vi "Dashboard Main.vi"() -> ()   [LabVIEW 2015]
uses:
  Camera Types.ctl
  <vilib>/Utility/miscctls.llb/LVRowAndColumnTypeDef.ctl
  <vilib>/event_ctls.llb/eventvkey.ctl
  <vilib>/Rock Robotics/WPI/Dashboard/WPI_DashboardLogging Global.vi
  <vilib>/Rock Robotics/Network Tables/NT Read Boolean.vi
  <vilib>/Utility/config.llb/Write Key (String).vi
  <vilib>/Utility/config.llb/Write Key (I32).vi
  <vilib>/Utility/config.llb/NI_LVConfig.lvlib
panel:
  in  "Input 2":u32
  in  "Input 1":u32
  out "Shooter Position":dbl
  out "Stowed Indicator":bool=TRUE
  out "Barf Shot Indicator":bool
  out "Far Shot Indicator":bool
  out "Close Shot Indicator":bool caption="Shooter Position"
  out "Yaw Indicator":bool
  out "Target Indicator":bool=TRUE
  out "Distance Indicator":bool=TRUE
  out "Angle Indicator":bool
  out "Ball Present Indicator":bool
  in  "TCP":refnum<k5>
  out "Camera IP":string="169.254.26.48"
  out "Image Message":string="Timeout in Camera Communications"
  in  "Dashboard Tab":T1(tab)=enum."Configuration"
  in  "Test Slider":dbl(slide) scale=0.0..100.0 scale format="%#_3g"
  in  "On/Off":bool caption="Solenoid"
  in  "Test Name":u16(ring) items=["Select the test to run..."]
  in  "Test Tree":string(tree)
  in  "Motor":cluster{"Value":dbl, "Enable":bool} {"Value" scale=-1.0..1.0 scale format="%#_3g"}
  out "Progress":T2 {"Test Progress" scale=0.0..100.0}
  in  "Rev/Fwd":cluster{"Forward":bool, "Reverse":bool}
  in  "Test Ring":u16(ring) items=["Monochrome", "Color"]
  out "Cmd Status":string
  in  "Execute Command":bool
  in  "Command Params":string[][](table)=[["No Input Parameters", "", ""]]
  in  "Command Selection":i32(listbox)
  in  "CheckList":i32(listbox)
  out "Tree":string(tree)
  in  "Tab Control":T3(tab)=enum."Load / Save"
  in  "Autonomous Mode":enum32{"0", "1", "2", "3"}(ring)
  in  "Position":i32(slide)=1 min=1 max=5 step=1 scale=1.0..5.0
  in  "Calibrate":bool
  out "Highest Score":dbl
  out "Distance (ft)":dbl
  in  "Reflective Tape Color":T4={"Hue"={112.792542, 147.565674}, "Sat"={128.447754, 128.447754}, "Val"={63.844784, 227.916416}} caption="Color Components" {"Val" scale=0.0..255.0; "Sat" scale=0.0..255.0; "Hue" scale=0.0..255.0 scale format="%#_3g"}
  in  "Test Mode":bool
  in  "Image":dbl=2.0 min=1.0 max=12.0 step=1.0
  in  "Min Score":dbl(slide) min=0.0 max=100.0 step=1.0 scale=0.0..100.0 scale format="%d%%"
  in  "Camera":T5=enum."MS HD3000 square"
  out "Targets":i32
  out "Vision Target Center":dbl=160.0 caption="Center (px)"
  in  "Y 2":dbl=60.0
  in  "X 2":dbl=100.0
  in  "Thickness 2":dbl=2.0
  in  "Y 1":dbl(slide)=126.0 scale=0.0..250.0
  in  "X 1":dbl(slide)=169.290323 scale=0.0..320.0
  in  "Show Center Line":bool
  in  "Close Shot Distance (ft)":dbl(slide)=9.0 min=0.0 max=10.0 scale=0.0..10.0
  in  "Far Shot Distance (ft)":dbl(slide)=10.5 min=0.0 max=10.0 scale=0.0..10.0
  in  "Close Shot":u32(colorbox)=16769066
  in  "Far Shot":u32(colorbox)=3538688
  in  "Show Target Box":bool=TRUE
  in  "Text Size":dbl
  in  "Too Far":u32(colorbox)=15663156
  in  "Show Crosshairs":bool=TRUE
  in  "Thickness 1":dbl=2.0
  out "Drivetrain Test Enabled":bool
  in  "D":dbl
  in  "I":dbl
  in  "P":dbl
  in  "Apply Test PID Values":bool
  in  "Px/Deg Conversion":dbl=0.1825 caption="1 px =                  degrees" min=0.0
  out "Difference (px)":dbl=-157.5
  out "Robot Center":dbl=317.5
  out "Target Align Center":dbl=160.0 caption="Target Center"
  out "Target Align Yaw Indicator":cluster{dbl, dbl}(knob) scale=-180.0..180.0
  out "Status":string
  out "INI File Path":path=path "Documents/FRC/DashboardSettings.ini"
  in  "Save Settings":bool
  out "File Created":bool
  out "Difference":dbl
  out "Starting Position":i32
  out "Autonomous Mode":enum32{"0", "1", "2", "3"}(ring)
  out "Intake":cluster{dbl, dbl}(knob) scale=0.0..5.0
  out "Time Remaining":dbl(slide)=-1.0 scale=-1.0..135.0 scale format="%#_6f"
  out "Battery Voltage":dbl(slide)=12.73828125 scale=0.012..12.0 scale format="%#_6f"
  out "Shooter":cluster{dbl, dbl}(knob) scale=0.0..5.0
  out "Yaw":cluster{dbl, dbl}(knob) scale=-180.0..180.0
  out "NT Connection":bool=TRUE
  in  "Camera Settings":T6={"Frame Rate"=30, "Compression"=30, "Size"=1} {"Frame Rate" scale=1.0..30.0; "Size" items=["640x480", "320x240", "160x120"]}
  out "Mode":T7(ring)
  in  "DB Camera Config":bool
  out "fps":dbl=30.150753768844222 format="%#.1g"
  out "Mbps":dbl=4.785927884198665 format="%#.1g"
  out "Mbps LED":bool=TRUE
  in  "Vision":u16(ring)=2 items=["Camera Off", "USB Camera SW", "USB Camera HW", "IP Camera", "Local"]
  in  "Rec Mode":enum32{"Stop", "Record", "Playback"}(radio)
  out "Background":bool=TRUE
  out "Distance":dbl
  out "Camera Image":T8(plugin-control)
  # "Close Shot"
  # "Far Shot"
  # "Target Box"
  # "Drivetrain Test PID Values"
  # "deg/px"
  # "Current Yaw"
  # "Target Yaw"
  # "* deg/px doesn't get saved, just initialized as default value"
  # "Setpoint"
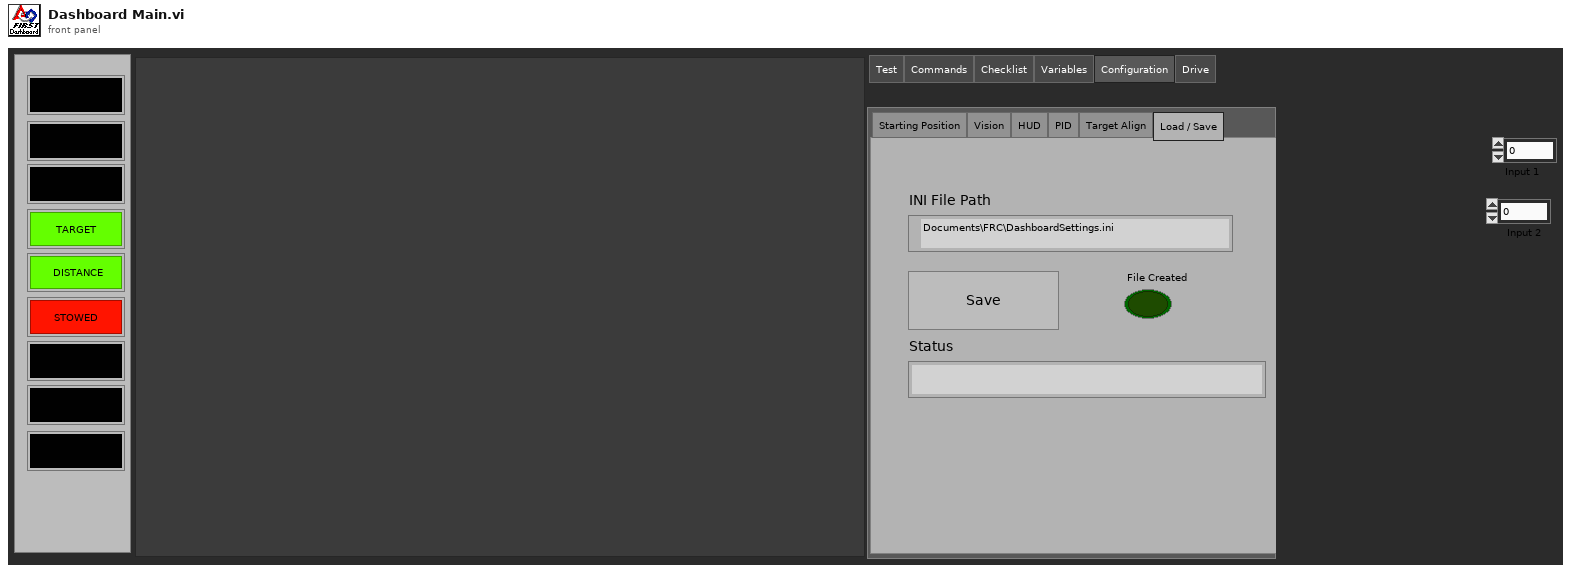
[diagram p1: front panel]
types:
  T1 = enum32{"Test", "Commands", "Checklist", "Variables", "Configuration", "Drive"}
  T2 = cluster{"Test Progress":u8, "Test Progress Text":string}
  T3 = enum32{"Starting Position", "Vision", "HUD", "PID", "Target Align", "Load / Save"}
  T4 = cluster{"Hue":cluster{dbl, dbl}, "Sat":cluster{dbl, dbl}, "Val":cluster{dbl, dbl}}
  T5 = typedef "Camera Types.ctl" = enum16{"206", "1011", "1013", "MS HD3000 square", "MS HD3000 640x480"}
  T6 = cluster{"Frame Rate":i32, "Compression":i32, "Size":u16}
  T7 = enum8{"Tele-Op Disabled", "Tele-Op Enabled", "Auto Disabled", "Auto Enabled", "Test Disabled", "Test Enabled", "Disconnected", "No Code", "E-Stop"}
  T8 = typedef "IMAQ Image.ctl" = refnum<image>
  T9 = typedef "Image Type" = u32
  T10 = cluster{"IDs":cluster{"RPC field ID":u16, "Unique ID":u16}, "String":string}
  T11 = cluster{"Camera Image":refnum<vi>, "Dashboard Tab":refnum<vi>, "Background":refnum<vi>, "Vision":refnum<vi>, "Rec Mode":refnum<vi>, "Test Slider":refnum<vi>, "On/Off ":refnum<vi>, "Test Ring":refnum<vi>, "Rev/Fwd":refnum<vi>, "Test Name":refnum<vi>, "Motor":refnum<vi>, "Progress":refnum<vi>, "CheckList":refnum<vi>, "Tree":refnum<vi>, "Test Tree":refnum<vi>, "Command Params":refnum<vi>, "Command Selection":refnum<vi>, "Execute Command":refnum<vi>, "Cmd Status":refnum<vi>}
  T12 = typedef "NI_LVConfig.lvlib/Config Data RefNum.ctl" = refnum<k1>
  T13 = cluster{"Error Strings":string, "Disable Counts":cluster{u16, u16}, "Rail Faults":cluster{u16, u16, u16}, "Robot IP":string, "DB Mode":u8, "Event Info":cluster{"Name":string, "Type":u8, "Number":u16, "Replay":u8}, "Camera Addr":string}
  T14 = cluster{"Storage":cluster{"Disk Free":u64, "RAM Block":u32, "RAM free":u32}, "CPU Utilization":cluster{"CPU % ISR":sgl, "CPU % Time Crit":sgl, "CPU % Timed Str":sgl, "CPU % High":sgl, "CPU % Above":sgl, "CPU % Normal":sgl, "CPU % Low":sgl}, "CAN":cluster{"% Bus Utilization":sgl, "Bus Off Cnt":u32, "TX_FIFO Full Cnt":u32, "Receive Error Cnt":u8, "Transmit Error Cnt":u8}, "HID":cluster{"HID Outputs":u32, "Rumble Low":u16, "Rumble High":u16}[]}
  T15 = cluster{"Status bits":cluster{"Test Mode":bool, "Autonomous":bool, "Enabled":bool, "Code Start":bool, "Brownout":bool, "Reserved 2":bool, "Reserved 3":bool, "E-Stop":bool}, "Code Trace":cluster{"Disabled":bool, "TeleOp":bool, "Auto":bool, "Test":bool}, "Controller Type":enum16{"unknown", "cRIO", "roboRio"}, "Code?":enum16{"unknown", "noCode", "code"}, "Battery V":dbl}
  T16 = cluster{"Control Bits":cluster{"TestMode":bool, "Autonomous":bool, "Enabled":bool, "FMS Present":bool, bool, bool, bool, "E-Stop":bool}, "Team Station ":u8, "Countdown":sgl, "Joystick Values":cluster{"Axes":dbl[], "Buttons":bool[], "POVs":i16[]}[]}
  T17 = cluster{"Operation":enum16{"Update", "Clear"}, "Color Box":u32}[]
  T18 = typedef "eventvkey.ctl" = enum16{"ASCII", "Enter", "Return", "Shift", "Ctrl", "Alt", "Cmd", "Opt", "Caps", "NumLock", "Clear", "Break", "Up", "Down", "Left", "Right", "Insert", "Delete", "Home", "End", "PageUp", "PageDown", "Escape", "Help", "Pause", "ScrollLock", "F1", "F2", "F3", "F4", "F5", "F6", "F7", "F8", "F9", "F10", "F11", "F12", "F13", "F14", "F15", "F16", "F17", "F18", "F19", "F20", "F21", "F22", "F23", "F24", "Play", "VolumeUp", "VolumeDown", "Mute", "Two Byte Char"}
  T19 = cluster{"Image Size":bool, "Image Type":bool, "Pixel Value":bool, "ROI Information":bool, "Zoom Factor":bool}
  T20 = enum8{"Enabled", "Disabled", "Disabled and Grayed Out"}
  T21 = cluster{"Operation":enum16{"Update", "Clear"}, "Color Box":u32}
  T22 = typedef "LVRowAndColumnTypeDef.ctl" = cluster{"Row":i32, "Column":i32}
  T23 = cluster{"Shift":bool, "Ctrl":bool, "Alt":bool, "Cmd":bool, "Opt":bool}
  T24 = cluster{"Hue Max":dbl, "Hue Min":dbl, "Sat Max":dbl, "Sat Min":dbl, "Val Max":dbl, "Val Min":dbl, "Far Shot Distance (ft)":dbl, "Close Shot Distance (ft)":dbl, "Thickness 1":dbl, "Input 1":dbl, "X 2":dbl, "Y 2":dbl, "Thickness 2":dbl, "Input 2":dbl, "X 1":dbl, "Y 1":dbl, "Min Score":dbl}
  T25 = cluster{cluster{dbl, dbl}, cluster{dbl, dbl}, cluster{dbl, dbl}}
  T26 = cluster{dbl, dbl, dbl, dbl, dbl, dbl, "Far Shot Distance (ft)":dbl, "Close Shot Distance (ft)":dbl, "X 1":dbl, "Y 1":dbl, "Thickness 1":dbl, "Input 1":u32, "X 2":dbl, "Y 2":dbl, "Thickness 2":dbl, "Input 2":u32, "Min Score":dbl}
  T27 = cluster{"Distance (ft)":dbl, "Center":cluster{dbl, dbl}, "Normalized Rect":cluster{"Left":dbl, "Top":dbl, " Right":dbl, "Bottom":dbl}}
  T28 = cluster{"Distance (ft)":dbl, "Center":cluster{dbl, dbl}, "Normalized Rect":cluster{"Numeric":dbl, "Numeric 2":dbl, "Numeric 3":dbl, "Numeric 5":dbl}}[]
  T29 = cluster{"Distance (ft)":dbl, "Center":cluster{dbl, dbl}, " Bounding Rect":cluster{"Left":dbl, "Top":dbl, " Right":dbl, "Bottom":dbl}}
  T30 = cluster{"Left":dbl, "Top":dbl, " Right":dbl, "Bottom":dbl}
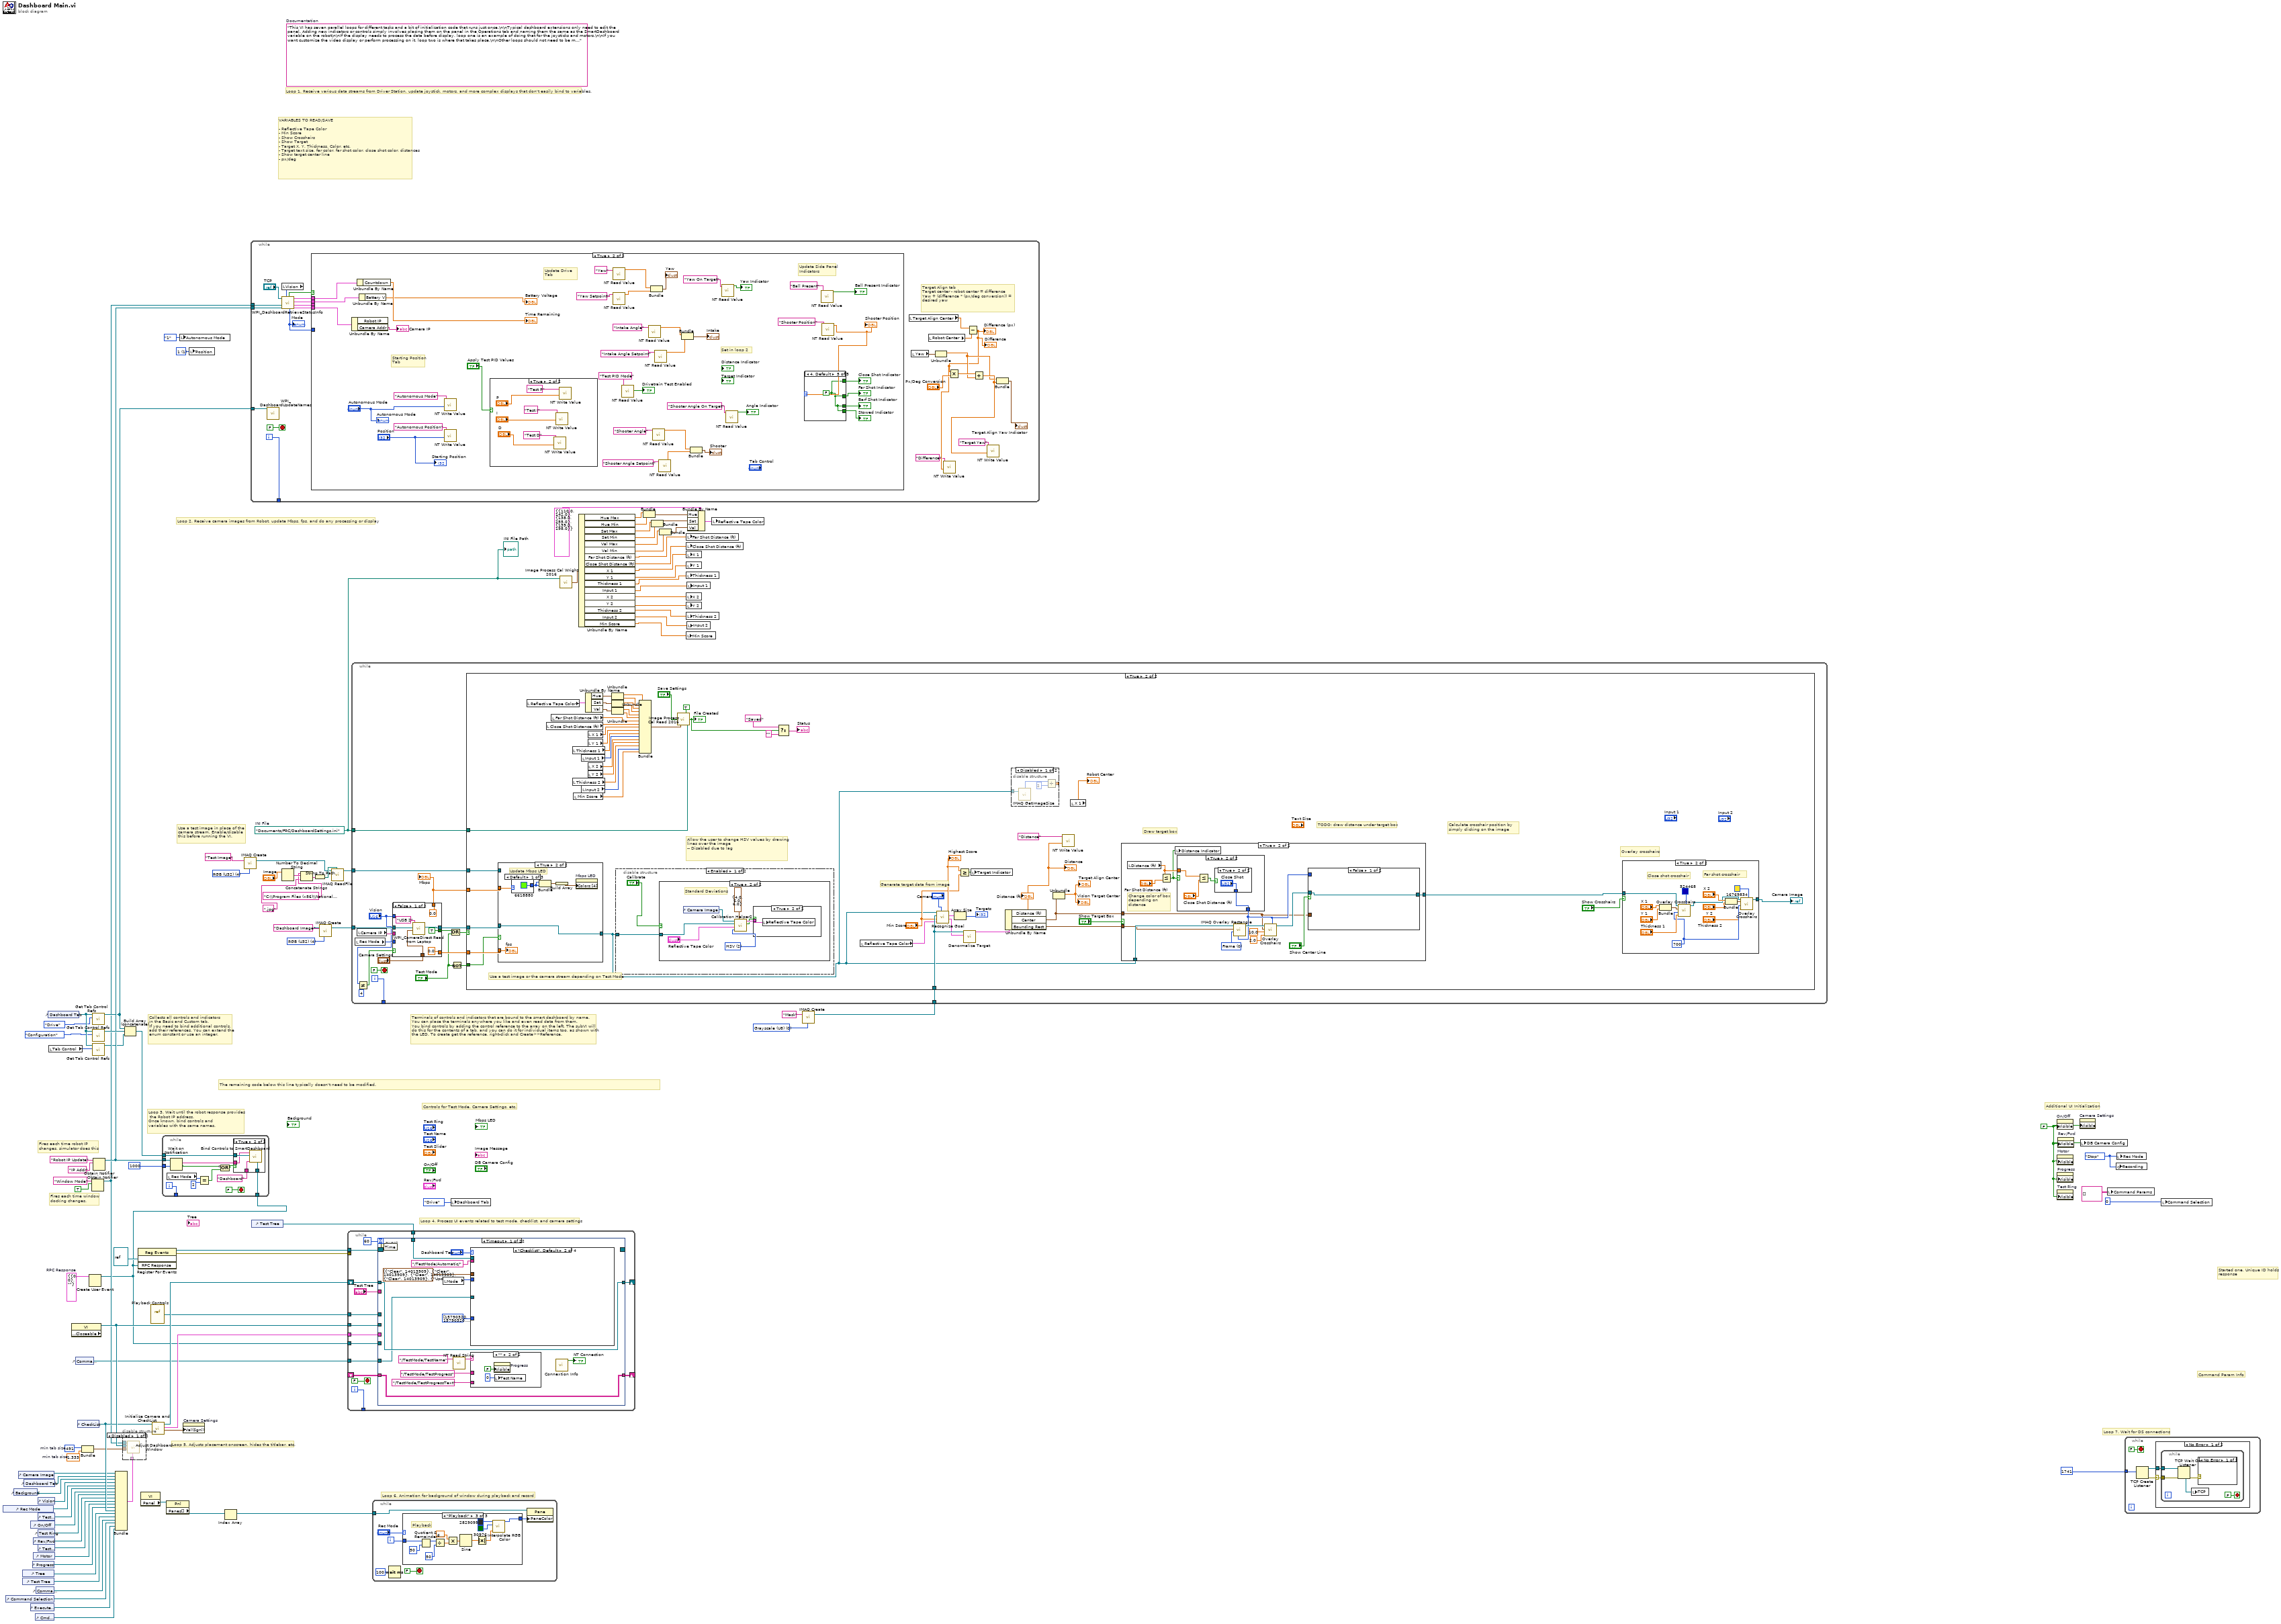
[diagram p0: block diagram]
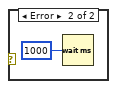
[diagram p4: hidden frame]
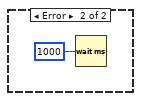
[diagram p5: hidden frame]
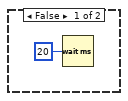
[diagram p6: hidden frame]
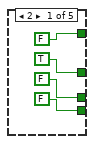
[diagram p8: hidden frame]
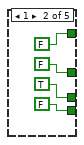
[diagram p9: hidden frame]
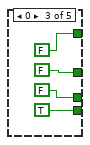
[diagram p10: hidden frame]
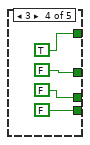
[diagram p11: hidden frame]
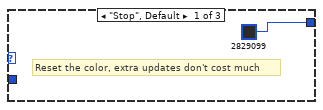
[diagram p12: hidden frame]
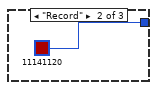
[diagram p13: hidden frame]
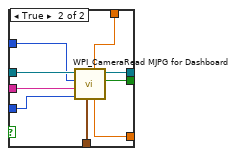
[diagram p14: hidden frame]
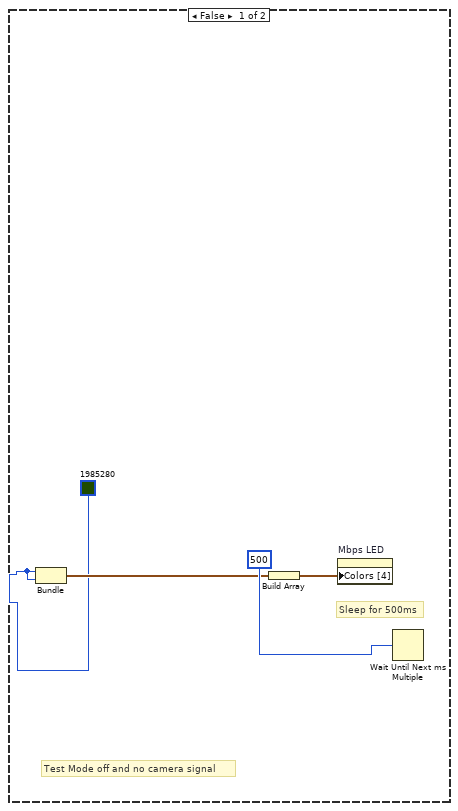
[diagram p15: hidden frame]
diagram:
  w1 = 1 items=["0", "1", "2", "3", "4", "5"] ("Position")
  w26 = 491  # min tab size
  w25 = 1.333  # min tab size
  w42 = path "Documents/FRC/DashboardSettings.ini"  # INI File
  w58 = T9 4 items=["Grayscale (U8)", "Grayscale (I16)", "Grayscale (SGL)", "Complex (CSG)", "RGB (U32)", "HSL (U32)", "RGB (U64)"] ("Image Type")
  w68 = T9 0 items=["Grayscale (U8)", "Grayscale (I16)", "Grayscale (SGL)", "Complex (CSG)", "RGB (U32)", "HSL (U32)", "RGB (U64)"] ("Image Type")
  w74 = T10 {"IDs"={"RPC field ID"=0, "Unique ID"=0}, "String"=""}  # RPC Response
  w84 = enum32{"Stop", "Record", "Playback"}."Stop" ("Rec Mode")
  w79 = FALSE ("Visible")
  (unwired) "This VI has seven parallel loops for different tasks and a bit of initialization code that runs just once.\n\nTypical dashboard extensions only need to edit the panel. Adding new indicators or controls simply involves placing them on the panel in the Operations tab and naming them the same as the SmartDashboard variable on the robot\n\nIf the display needs to process the data before display, loop one is an example of doing that for the joysticks and motors.\n\nIf you want customize the video display or perform processing on it, loop two is where that takes place.\n\nOther loops should not need to be modified. They are pretty standard, and document the task they perform."  # Documentation
  w101 = T9 4 items=["Grayscale (U8)", "Grayscale (I16)", "Grayscale (SGL)", "Complex (CSG)", "RGB (U32)", "HSL (U32)", "RGB (U64)"] ("Image Type")
  # "Loop 3. Wait until the robot response provides\n the Robot IP address.\nOnce known, bind controls and\nvariables with the same names."
  # "VARIABLES TO READ/SAVE\n\n- Reflective Tape Color\n- Min Score\n- Show Crosshairs\n- Show Target\n- Target X, Y, Thickness, Color, etc.\n- Target text size, far color, far shot color, close shot color, distances\n- Show target center line\n- px/deg"
  # "Use a test image in place of the camera stream. Enable/disable this before running the VI."
  # "Command Param Info"
  # "Started one, Unique ID holds\nresponse"
  # "Loop 7. Wait for DS connections"
  # "Controls for Test Mode, Camera Settings, etc."
  # "Additional UI Initialization"
  # "Loop 6. Animation for background of window during playback and record"
  # "Fires each time robot IP\nchanges, simulator does this"
  # "Fires each time window\ndocking changes."
  # "Collects all controls and indicators\nin the Basic and Custom tab.\nIf you need to bind additional controls,\nadd their references. You can extend the\nenum constant or use an integer."
  # "The remaining code below this line typically doesn't need to be modified."
  # "Loop 4. Process UI events related to test mode, checklist, and camera settings"
  # "Terminals of controls and indicators that are bound to the smart dashboard by name.\nYou can place the terminals anywhere you like and even read data from them.\nYou bind controls by adding the control reference to the array on the left. The subVI will\ndo this for the contents of a tab, and you can do it for individual items too, as shown with\nthe LED. To create get the reference, right-click and Create>>Reference."
  # "Loop 5. Adjusts placement onscreen, hides the titlebar, etc."
  # "Loop 1. Receive various data streams from Driver Station, update joystick, motors, and more complex displays that don't easily bind to variables."
  # "Loop 2. Receive camera images from Robot, update Mbps, fps, and do any processing or display"
  n1 = control-ref of="Rec Mode"() -> (w18:refnum<vi>)
  n2 = control-ref of="Command Selection"() -> (w10:refnum<vi>)
  n3 = control-ref of="Background"() -> (w8:refnum<vi>)
  n4 = control-ref of="Camera Image"() -> (w29:refnum<vi>)
  n5 = control-ref of="Tree"() -> (w22:refnum<vi>)
  n6 = control-ref of="Test Tree"() -> (w21:refnum<vi>)
  n7 = control-ref of="Dashboard Tab"() -> (w28:refnum<vi>)
  n8 = control-ref of="Execute Command"() -> (w11:refnum<vi>)
  n9 = control-ref of="On/Off"() -> (w16:refnum<vi>)
  n10 = control-ref of="Progress"() -> (w13:refnum<vi>)
  n11 = control-ref of="Rev/Fwd"() -> (w14:refnum<vi>)
  n12 = control-ref of="Motor"() -> (w19:refnum<vi>)
  n13 = control-ref of="Cmd Status"() -> (w9:refnum<vi>)
  n14 = control-ref of="Command Params"() -> (w12:refnum<vi>)
  n15 = control-ref of="Test Slider"() -> (w17:refnum<vi>)
  n16 = control-ref of="Vision"() -> (w27:refnum<vi>)
  n17 = control-ref of="Test Ring"() -> (w15:refnum<vi>)
  n18 = control-ref of="Test Name"() -> (w20:refnum<vi>)
  n19 = control-ref of="Dashboard Tab"() -> (w6:refnum<vi>)
  n20 = local read "Tab Control"() -> (w5:T3)
  n21 = property class="VI" props=["Front Panel.Closeable"]() -> (reference out=w83:refnum<vi>)  [unwired: 2 in, 2 out]
  n22 = control-ref of="Command Params"() -> (w70:refnum<vi>)
  n23 = control-ref of="CheckList"() -> (w80:refnum<vi>)
  n24 = Bundle("min tab size"=w26, "min tab size"=w25) -> (w24:cluster{"min tab size":i32, "min tab size":dbl})  [unwired: 1 in]
  n25 = Create User Event(user event datatype=w74) -> (user event=w71:refnum<user-event>)  [unwired: 1 in, 1 out]
  n26 = Obtain Notifier(name (unnamed)="Window Mode", notification data type=TRUE) -> (notifier out=w76:refnum<notifier>)  [unwired: 2 in, 2 out]
  n27 = call <vilib>:"Get Tab Control Refs.vi"("Page Index"=T1."Drive" ("Dashboard Tab"), "TabControl in"=w6) -> ("ControlsOnPage"=w77:refnum<vi>[])  [unwired: 9 in]
  n28 = call <vilib>:"Get Tab Control Refs.vi"("Page Index"=T1."Configuration" ("Dashboard Tab"), "TabControl in"=w6) -> ("ControlsOnPage"=w82:refnum<vi>[])  [unwired: 9 in]
  n29 = call <vilib>:"Get Tab Control Refs.vi"("Page Index"=w5, "TabControl in"=w6) -> ("ControlsOnPage"=w7:refnum<vi>[])  [unwired: 9 in]
  n30 = Obtain Notifier(name (unnamed)="Robot IP Update", notification data type="IP Addr" ("name (unnamed)")) -> (notifier out=w78:refnum<notifier>)  [unwired: 2 in, 2 out]
  n31 = Bundle("Camera Image"=w29, "Dashboard Tab"=w28, "Background"=w8, "Vision"=w27, "Rec Mode"=w18, "Test Slider"=w17, "On/Off"=w16, "Test Ring"=w15, "Rev/Fwd"=w14, "Test Name"=w20, "Motor"=w19, "Progress"=w13, "CheckList"=w80, "Tree"=w22, "Test Tree"=w21, "Command Params"=w12, "Command Selection"=w10, "Execute Command"=w11, "Cmd Status"=w9) -> (w23:T11)  [unwired: 1 in]
  n32 = disable-structure shown="Disabled" {
    disable-tunnel: w83 -> [w105 _]
    disable-tunnel: w76 -> [w104 _]
    disable-tunnel: w24 -> [w103 _]
    disable-tunnel: w23 -> [w102 _]
    frame Disabled {
      n33 = call "Adjust Dashboard Window.vi"("Sizing Refnums"=w102, "Size Constraints"=w103, "VI"=w105, "WIn Mode"=w104) -> ()  [unwired: 8 in]
    }
    frame Enabled {
    }
  }
  n34 = Build Array (concatenate)(w77, w82, w7) -> (w81:refnum<vi>[])
  n35 = register-events(refnum<vi> refnum, w71) -> (reference out=w87:refnum<event-registration>, error out=w86:errorcluster)  [unwired: 2 in]
  n36 = property class="VI"() -> ("Panel"=w90:refnum<vi>)  [unwired: 2 in, 2 out]
  n37 = vi-ref "Playback Controls.vi"() -> (w88:refnum<vi>)
  n38 = call "Initialize Camera and CheckList.vi"("ListBox in"=w80) -> ("Cluster"=w94:cluster{"value":i32, "value":i32, "index":i32}, "Array"=w95:cluster{string[]}[], "File Refnum"=w93:T12)  [unwired: 8 in]
  n39 = while {
    tunnel: w81 -> [w118]
    tunnel: w78 -> [w116]
    tunnel: [w114] -> _
    tunnel: u32 1000 ("milliseconds to wait") -> [w113]
    tunnel: w71 -> [w106]
    i -> [w114]
    stop <- FALSE stop-if-true
    n40 = local read "Rec Mode"() -> (w109:enum32{"Stop", "Record", "Playback"})
    n41 = Wait on Notification(notifier=w116, timeout in ms (-1)=w113) -> (notification=w115:string, timed out?=w111:bool)  [unwired: 2 in, 2 out]
    n42 = Equal?(x=w109, y=u16 2 ("Rec Mode")) -> (x = y?=w110:bool)
    n43 = Compound Arithmetic op=OR(invert w111, w110) -> (w112:bool)
    n44 = case shown="True" w112 {
      tunnel: w118 -> [_ w122]
      tunnel: w115 -> [_ w121]
      tunnel: "Dashboard" -> [_ w120]
      tunnel: w106 -> [_ w119]
      frame False {
      }
      frame True {
        n45 = call <vilib>:"Bind Controls to SmartDashboard.vi"("RPC ref"=w119, "Client Name"=w120, "Bound Control Refs"=w122, "Server IP Address"=w121) -> ()  [unwired: 8 in]
      }
    }
  }
  n46 = property class="Pnl"(reference=w90) -> ("Panes[]"=w91:refnum<vi>[])  [unwired: 1 in, 2 out]
  n47 = local write "Autonomous Mode"(enum32{"0", "1", "2", "3"}."1" ("Autonomous Mode")) -> ()
  n48 = property on="Camera Settings" class="Clust (strict)"("Val(Sgnl)"=w94) -> ()  [unwired: 2 in, 2 out]
  n49 = local write "Position"(w1) -> ()
  n50 = Index Array(array=w91) -> (element=w89:refnum<vi>)  [unwired: 1 in]
  n51 = call "IMAQ Create"("Image Name"="Test Image", "Image Type"=w58) -> ("New Image"=w56:T8)  [unwired: 2 in, 2 out]
  n52 = while {
    tunnel: [w145] -> _
    tunnel: w78 -> [w139]
    tunnel: w77 -> [w138]
    tunnel: w76 -> [w134]
    i -> [w145]
    stop <- FALSE stop-if-true
    # "Target Align tab\nTarget center - robot center = difference\nYaw + (difference * (px/deg conversion)) = desired yaw"
    n53 = call <vilib>:"WPI_DashboardUpdateNames.vi"("Controls on Tab"=w138) -> ()  [unwired: 11 in]
    n54 = local read "Vision"() -> (w136:u16)
    n55 = call <vilib>:"WPI_DashboardRetrieveStatusInfo.vi"("Vision"=w136, "Binding Refnum"=w139, "Window Mode Notifier"=w134, "TCP Cnx"="TCP") -> ("Power and Errors"=w140:T13, "Robot Metrics"=w143:T14, "Status Info"=w144:T15, "Control Info"=w141:T16, "Robot Mode"=w137:T7, "Process?"=w142:bool)  [unwired: 2 in]
    "Mode" <- w137
    n56 = case shown="True" w142 {
      tunnel: w144 -> [_ w187]
      tunnel: w143 -> [_ _]
      tunnel: w141 -> [_ w186]
      tunnel: w140 -> [_ w185]
      tunnel: w137 -> [_ _]
      frame False {
        n57 = Wait (ms)(milliseconds to wait=u32 20) -> ()  [unwired: 1 out]
      }
      frame True {
        # "Set in loop 2"
        # "Starting Position Tab"
        # "Update Side Panel Indicators"
        # "Update Drive Tab"
        n58 = Unbundle By Name(w185) -> ("Camera Addr"=→"Camera IP":string)  [unwired: 1 out]
        n59 = Unbundle By Name(w186) -> ("Countdown"=→"Time Remaining":sgl)
        n60 = Unbundle By Name(w187) -> ("Battery V"=→"Battery Voltage":dbl)
        n61 = call-poly <vilib>:"NT Write Value.vi"("Numeric"="Autonomous Mode", "Name"="Autonomous Mode") -> ()  [unwired: 9 in, 1 out]
        n62 = call-poly <vilib>:"NT Write Value.vi"("Numeric"="Position", "Name"="Autonomous Position") -> ()  [unwired: 9 in, 1 out]
        n63 = case shown="True" "Apply Test PID Values" {
          frame False {
          }
          frame True {
            n64 = call-poly <vilib>:"NT Write Value.vi"("Numeric"="D", "Name"="Test D") -> ()  [unwired: 9 in, 1 out]
            n65 = call-poly <vilib>:"NT Write Value.vi"("Numeric"="I", "Name"="Test I") -> ()  [unwired: 9 in, 1 out]
            n66 = call-poly <vilib>:"NT Write Value.vi"("Numeric"="P", "Name"="Test P") -> ()  [unwired: 9 in, 1 out]
          }
        }
        n67 = call-poly <vilib>:"NT Read Value.vi"("Name"="Yaw") -> ("Numeric"=w180:dbl)  [unwired: 9 in, 1 out]
        n68 = call-poly <vilib>:"NT Read Value.vi"("Name"="Yaw Setpoint") -> ("Numeric"=w179:dbl)  [unwired: 9 in, 1 out]
        n69 = call-poly <vilib>:"NT Read Value.vi"("Name"="Test PID Mode") -> ("Boolean"=→"Drivetrain Test Enabled":bool)  [unwired: 9 in, 1 out]
        n70 = call-poly <vilib>:"NT Read Value.vi"("Name"="Intake Angle") -> ("Numeric"=w157:dbl)  [unwired: 9 in, 1 out]
        n71 = Bundle("Numeric"=w180, "Numeric"=w179) -> (→"Yaw":cluster{"Numeric":dbl, "Numeric":dbl})  [unwired: 1 in]
        n72 = call-poly <vilib>:"NT Read Value.vi"("Name"="Shooter Angle") -> ("Numeric"=w174:dbl)  [unwired: 9 in, 1 out]
        n73 = call-poly <vilib>:"NT Read Value.vi"("Name"="Intake Angle Setpoint") -> ("Numeric"=w156:dbl)  [unwired: 9 in, 1 out]
        n74 = call-poly <vilib>:"NT Read Value.vi"("Name"="Shooter Angle Setpoint") -> ("Numeric"=w176:dbl)  [unwired: 9 in, 1 out]
        n75 = Bundle("Numeric"=w157, "Numeric"=w156) -> (→"Intake":cluster{"Numeric":dbl, "Numeric":dbl})  [unwired: 1 in]
        n76 = Bundle("Numeric"=w174, "Numeric"=w176) -> (→"Shooter":cluster{"Numeric":dbl, "Numeric":dbl})  [unwired: 1 in]
        n77 = call-poly <vilib>:"NT Read Value.vi"("Name"="Yaw On Target") -> ("Boolean"=→"Yaw Indicator":bool)  [unwired: 9 in, 1 out]
        n78 = call-poly <vilib>:"NT Read Value.vi"("Name"="Shooter Angle On Target") -> ("Boolean"=→"Angle Indicator":bool)  [unwired: 9 in, 1 out]
        n79 = call-poly <vilib>:"NT Read Value.vi"("Name"="Ball Present") -> ("Boolean"=→"Ball Present Indicator":bool)  [unwired: 9 in, 1 out]
        n80 = call-poly <vilib>:"NT Read Value.vi"("Name"="Shooter Position") -> ("Numeric"=w170:dbl)  [unwired: 9 in, 1 out]
        "Shooter Position" <- w170
        n81 = case shown="4, Default" w170 {
          tunnel: [FALSE FALSE FALSE TRUE w210] -> w169
          tunnel: [TRUE FALSE FALSE FALSE w210] -> w168
          tunnel: [FALSE TRUE FALSE FALSE w210] -> w167
          tunnel: [FALSE FALSE TRUE FALSE w210] -> w166
          frame 2 {
          }
          frame 1 {
          }
          frame 0 {
          }
          frame 3 {
          }
          frame 4, Default {
            w210 = FALSE
          }
        }
        "Stowed Indicator" <- w166
        "Close Shot Indicator" <- w169
        "Far Shot Indicator" <- w168
        "Barf Shot Indicator" <- w167
        "Autonomous Mode" <- "Autonomous Mode"
        "Starting Position" <- "Position"
      }
    }
    n82 = local read "Target Align Center"() -> (w130:dbl)
    n83 = local read "Yaw"() -> (w126:cluster{dbl, dbl})
    n84 = local read "Robot Center"() -> (w133:dbl)
    n85 = Unbundle(w126) -> (w125:dbl)  [unwired: 1 out]
    n86 = Subtract(x=w130, y=w133) -> (x-y=w124:dbl)
    "Difference (px)" <- w124
    "Difference" <- w124
    n87 = call-poly <vilib>:"NT Write Value.vi"("Numeric"=w124, "Name"="Difference") -> ()  [unwired: 9 in, 1 out]
    n88 = Multiply(x=w124, y="Px/Deg Conversion") -> (x*y=w131:dbl)
    n89 = Add(x=w131, y=w125) -> (x+y=w129:dbl)
    n90 = call-poly <vilib>:"NT Write Value.vi"("Numeric"=w129, "Name"="Target Yaw") -> ()  [unwired: 9 in, 1 out]
    n91 = Bundle(w125, w129) -> (→"Target Align Yaw Indicator":cluster{dbl, dbl})  [unwired: 1 in]
  }
  n92 = control-ref of="Test Tree"() -> (w92:refnum<vi>)
  n93 = Number To Decimal String(number="Image") -> (decimal integer string=w63:string)  [unwired: 1 in]
  n94 = Concatenate Strings("C:\\Program Files (x86)\\National Instruments\\LabVIEW 2015\\examples\\FRC\\roboRIO\\Vision\\2016 Vision Example\\Sample Images\\Real Tower\\image", w63, ".jpg" ("string")) -> (w64:string)
  n95 = String To Path(string=w64) -> (path=w59:path)
  n96 = call "IMAQ Create"("Image Name"="Dashboard Image", "Image Type"=w101) -> ("New Image"=w65:T8)  [unwired: 2 in, 2 out]
  n97 = call "IMAQ ReadFile"("File Path"=w59, "Image"=w56) -> ("Image Out"=w55:T8)  [unwired: 5 in, 4 out]
  n98 = while {
    tunnel: w95 -> [w222]
    shift-right: [w221] -> _
    shift-left: w93 -> [w220]
    tunnel: [w219] -> _
    tunnel: w92 -> [w218]
    tunnel: w88 -> [w217]
    tunnel: w87 -> [w216]
    tunnel: w86 -> [_]
    tunnel: w83 -> [w215]
    tunnel: w71 -> [w214]
    tunnel: w70 -> [w213]
    shift-right: [w212] -> _
    shift-left: _ -> [w211]
    i -> [w219]
    stop <- FALSE stop-if-true
    n99 = event shown="[0] Timeout" {
      selector: w216 -> [_ _ _ _ _ _ _ _ _ _ _ _ _ _ _ _ _ _ _ _ _ _]
      dyn-events: [_ _ _ _ _ _ _ _ _ _ _ _ _ _ _ _ w523 _ _ _ _ _] -> _
      timeout: u32 60 ("milliseconds to wait") -> [_ _ _ _ _ _ _ _ _ _ _ _ _ _ _ _ _ _ _ _ _ _]
      tunnel: w218 -> [w235 _ _ _ _ _ _ _ _ _ _ _ _ _ _ _ _ _ _ _ _ _]
      tunnel: "Test Tree" -> [_ _ _ _ _ _ _ _ _ _ _ w486 w495 w498 w503 w512 _ _ _ _ _ _]
      tunnel: w222 -> [_ w273 _ _ _ _ _ _ _ w448 w479 _ _ _ _ _ _ _ _ _ _ _]
      tunnel: [w232 w272 w376 w382 w394 w406 w414 w420 w433 w447 w472 w485 w493 w497 w502 w511 w525 w541 w543 w551 w562 w567] -> w221
      tunnel: w220 -> [w232 w272 w376 w382 w394 w406 w414 w420 w433 w446 w472 w485 w493 w497 w502 w511 w525 w541 w543 w551 w562 w567]
      tunnel: w217 -> [_ _ _ _ _ _ _ _ _ _ _ _ _ _ _ _ w526 _ w546 _ _ _]
      tunnel: w215 -> [_ _ _ _ _ _ _ _ _ _ _ _ _ _ _ _ w521 _ _ _ _ _]
      tunnel: w214 -> [_ _ _ _ _ _ _ _ _ _ _ _ _ _ _ _ w517 _ _ _ _ _]
      tunnel: w213 -> [w227 _ _ _ w392 _ _ _ _ _ _ _ _ _ _ _ _ _ _ _ _ _]
      tunnel: [w226 w271 w375 w381 w390 w400 w411 w419 w432 w445 w471 w484 w492 w496 w501 w510 w516 w539 w542 w547 w555 w568] -> w212
      tunnel: w211 -> [w226 w271 w375 w381 w390 _ _ w419 w432 w445 w471 w484 w492 w496 w501 w510 w516 w539 w542 w547 w555 w568]
      event Timeout {
        n100 = event-data() -> ()  [unwired: 1 in, 1 out]
        n101 = local read "Mode"() -> (w229:T7)
        n102 = call <vilib>:"NT Read String.vi"("Name"="/TestMode/TestName") -> ("String"=w238:string)  [unwired: 9 in, 1 out]
        n103 = case shown="\"Checklist\", Default" "Dashboard Tab" {
          tunnel: w235 -> [w249 _ _ _]
          tunnel: "/TestMode/Automatic/" ("Name Pattern") -> [w248 _ _ _]
          tunnel: T17 [{"Operation"=enum."Clear", "Color Box"=14013909}, {"Operation"=enum."Clear", "Color Box"=14013909}, {"Operation"=enum."Clear", "Color Box"=14013909}, {"Operation"=enum."Clear", "Color Box"=14013909}, {"Operation"=enum."Update", "Color Box"=14013909}, {"Operation"=enum."Update", "Color Box"=16777215}, {"Operation"=enum."Clear", "Color Box"=14013909}, {"Operation"=enum."Clear", "Color Box"=14013909}, {"Operation"=enum."Clear", "Color Box"=14013909}] -> [w241 _ _ w258]
          tunnel: w229 -> [w240 _ _ w257]
          tunnel: u32[] [15790320, 15790320, 15790320, 15790320, 16777215, 16777215, 15790320, 15790320, 15790320] -> [_ _ _ w263]
          tunnel: w227 -> [_ _ _ w251]
          frame "Test" {
            w247 = -2 ("Active Item:Row Number")
            n104 = Index Array(array=w241, index=w240) -> (element=w242:T21)
            n105 = Unbundle(w242) -> ("Operation"=w243:enum16{"Update", "Clear"}, "Color Box"=w244:u32)
            n106 = call <vilib>:"NT Read and Format Entries as Tree.vi"("Operation"=w243, "Name Pattern"=w248, "Tree Refnum"=w249) -> ()  [unwired: 7 in, 2 out]
            n107 = property on="Test Tree" class="Tree (strict)"("Active Item Row Number"=w247, "ActiveColNum"=w247, "CellBG"=w244, "Active Item Row Number"=-1 ("Active Item:Row Number"), "CellBG"=u32 5789784 ("Color Box")) -> ()  [unwired: 2 in, 2 out]
          }
          frame "Checklist", Default {
          }
          frame "Variables" {
            n108 = control-ref of="Tree"() -> (w250:refnum<vi>)
            n109 = call <vilib>:"NT Read and Format Entries as Tree.vi"("Tree Refnum"=w250) -> ()  [unwired: 9 in, 2 out]
          }
          frame "Commands" {
            w259 = u32 5789784 ("Color Box")
            w260 = T22 {"Row"=-1, "Column"=-2} ("Active Cell:Active Cell")
            w262 = T22 {"Row"=-2, "Column"=-2} ("Active Cell:Active Cell")
            n110 = Index Array(array=w263, index=w257) -> (element=w261:u32)
            n111 = Index Array(array=w258, index=w257) -> (element=w256:T21)
            n112 = Unbundle(w256) -> ("Operation"=w255:enum16{"Update", "Clear"})  [unwired: 1 out]
            n113 = local read "Command Selection"() -> (w254:i32)
            n114 = property on="Command Selection" class="MCListbox (strict)"("ActiveCell"=w262, "CellBG"=w261, "ActiveCell"=w260, "CellBG"=w259) -> ()  [unwired: 2 in, 2 out]
            n115 = call <vilib>:"WPI_DashboardUpdate RPC Info.vi"("Operation"=w255) -> ("update"=w253:bool, "commands"=w252:string[][])  [unwired: 9 in]
            n116 = property on="Command Selection" class="MCListbox (strict)"("ItemNames"=w252) -> ()  [unwired: 2 in, 2 out]
            n117 = property on="Command Params" class="Tbl (strict)"("Active Cell"=w262, "Cell BG Color"=w261, "Active Cell"=w260, "Cell BG Color"=w259) -> ()  [unwired: 2 in, 2 out]
            n118 = call <vilib>:"WPI_DashboardUpdate Command Params.vi"("Update"=w253, "NewVal"=w254, "Commands"=w252, "Param Tbl"=w251) -> ()  [unwired: 7 in, 1 out]
          }
        }
        n119 = case shown="\"\"" w238 {
          tunnel: "/TestMode/TestProgress" ("Name") -> [w265 _]
          tunnel: "/TestMode/TestProgressText" ("Name") -> [w264 _]
          frame Default {
            n120 = call <vilib>:"NT Read Number.vi"("Name"=w265) -> ("Numeric"=w266:dbl)  [unwired: 9 in, 1 out]
            n121 = call <vilib>:"NT Read String.vi"("Name"=w264) -> ("String"=w267:string)  [unwired: 9 in, 1 out]
            n122 = Bundle("Numeric"=w266, "String"=w267) -> (→"Progress":cluster{"Numeric":dbl, "String":string})  [unwired: 1 in]
          }
          frame "" {
            n123 = property on="Progress" class="Clust (strict)"("Visible"=FALSE) -> ()  [unwired: 2 in, 2 out]
            n124 = local write "Test Name"(u16 0) -> ()
          }
        }
        n125 = call <vilib>:"Connextion Info.vi"() -> ("Connected"=→"NT Connection":bool)  [unwired: 10 in, 1 out]
      }
      event "Test Tree": Value Change {
        # "Show appropriate\ncontrols"
        n126 = event-data() -> ("CtlRef"=w276:refnum<vi>, "NewVal"=w274:string)  [unwired: 1 in]
        n127 = call <vilib>:"WPI_UtilitiesGetTreeIOName.vi"("NewVal"=w274, "TreeControl in"=w276) -> ("I/O Name"=w277:string)  [unwired: 9 in]
        n128 = case shown="\"Relay\", \"Solenoid\"" w277 {
          selector: w277 -> [_ w284 _ w306 w315 _]
          tunnel: w274 -> [_ _ w303 w305 _ w322]
          tunnel: w273 -> [_ _ _ _ _ w321]
          frame Default {
            w279 = FALSE ("Visible")
            w278 = FALSE ("Visible")
            n129 = property on="Motor" class="Clust (strict)"("Visible"=w278) -> ()  [unwired: 2 in, 2 out]
            n130 = property on="Test Ring" class="Ring (strict)"("Visible"=w278) -> ()  [unwired: 2 in, 2 out]
            n131 = property on="Rev/Fwd" class="Clust (strict)"("Visible"=w279) -> ()  [unwired: 2 in, 2 out]
            n132 = property on="On/Off" class="Bool (strict)"("Visible"=w279) -> ()  [unwired: 2 in, 2 out]
            n133 = property on="Test Slider" class="Slide (strict)"("Visible"=w279) -> ()  [unwired: 2 in, 2 out]
          }
          frame "Analog Out", "Motor", "PWM" {
            w285 = FALSE ("Visible")
            n134 = case shown="\"Analog Out\"" w284 {
              tunnel: [1.0 ("Value") -1.0 ("Value") 0.0 ("Value")] -> w283
              tunnel: [255.0 ("Value") 1.0 ("Value") 5.0 ("Value")] -> w282
              tunnel: [128.0 ("Value") 0.0 ("Value") 0.0 ("Value")] -> w281
              tunnel: [64.0 ("Value") 0.5 ("Value") 1.0 ("Value")] -> w280
              frame "PWM" {
              }
              frame "Motor", Default {
              }
              frame "Analog Out" {
              }
            }
            n135 = property on="Motor" class="Clust (strict)"("Visible"=TRUE) -> ()  [unwired: 2 in, 2 out]
            n136 = property on="Value" class="Slide (strict)"("Value"=w281, "Scale.Minimum"=w283, "Scale.Maximum"=w282, "Scale.Increment"=w280) -> ()  [unwired: 2 in, 2 out]
            n137 = property on="On/Off" class="Bool (strict)"("Visible"=w285) -> ()  [unwired: 2 in, 2 out]
            n138 = property on="Test Slider" class="Slide (strict)"("Visible"=w285) -> ()  [unwired: 2 in, 2 out]
            n139 = property on="Test Ring" class="Ring (strict)"("Visible"=w285) -> ()  [unwired: 2 in, 2 out]
            n140 = property on="Rev/Fwd" class="Clust (strict)"("Visible"=w285) -> ()  [unwired: 2 in, 2 out]
          }
          frame "Servo" {
            w301 = FALSE ("Visible")
            n141 = call <vilib>:"NT Read Number.vi"("Name"=w303) -> ("Numeric"=w302:dbl)  [unwired: 9 in, 1 out]
            n142 = property on="Test Slider" class="Slide (strict)"("Visible"=TRUE, "Scale.Maximum"=170.0 ("Scale.Range:Maximum")) -> ()  [unwired: 2 in, 2 out]
            n143 = local write "Test Slider"(w302) -> ()
            n144 = property on="Motor" class="Clust (strict)"("Visible"=w301) -> ()  [unwired: 2 in, 2 out]
            n145 = property on="Rev/Fwd" class="Clust (strict)"("Visible"=w301) -> ()  [unwired: 2 in, 2 out]
            n146 = property on="On/Off" class="Bool (strict)"("Visible"=w301) -> ()  [unwired: 2 in, 2 out]
            n147 = property on="Test Ring" class="Ring (strict)"("Visible"=w301) -> ()  [unwired: 2 in, 2 out]
          }
          frame "Relay", "Solenoid" {
            w304 = FALSE ("Visible")
            n148 = property on="Motor" class="Clust (strict)"("Visible"=w304) -> ()  [unwired: 2 in, 2 out]
            n149 = property on="Test Slider" class="Slide (strict)"("Visible"=w304) -> ()  [unwired: 2 in, 2 out]
            n150 = Search and Replace String(input string=w305, search string="/Value  **", replace string="/Direction") -> (result string=w311:string)  [unwired: 5 in, 3 out]
            n151 = property on="Test Ring" class="Ring (strict)"("Visible"=w304) -> ()  [unwired: 2 in, 2 out]
            n152 = call <vilib>:"NT Read String.vi"("Name"=w311) -> ("String"=w309:string)  [unwired: 9 in, 1 out]
            n153 = Equal?(x="Both directions", y=w309) -> (x = y?=w307:bool)
            n154 = Not(x=w307) -> (.not. x?=w308:bool)
            n155 = property on="Rev/Fwd" class="Clust (strict)"("Visible"=w307) -> ()  [unwired: 2 in, 2 out]
            n156 = property on="On/Off" class="Bool (strict)"("Visible"=w308, "Caption.Text"=w306) -> ()  [unwired: 2 in, 2 out]
          }
          frame "Compressor", "Digital Out" {
            w314 = FALSE ("Visible")
            # "Get direction and finish"
            n157 = property on="Motor" class="Clust (strict)"("Visible"=w314) -> ()  [unwired: 2 in, 2 out]
            n158 = property on="Test Slider" class="Slide (strict)"("Visible"=w314) -> ()  [unwired: 2 in, 2 out]
            n159 = property on="Test Ring" class="Ring (strict)"("Visible"=w314) -> ()  [unwired: 2 in, 2 out]
            n160 = property on="On/Off" class="Bool (strict)"("Visible"=TRUE, "Caption.Text"=w315) -> ()  [unwired: 2 in, 2 out]
            n161 = property on="Rev/Fwd" class="Clust (strict)"("Visible"=FALSE) -> ()  [unwired: 2 in, 2 out]
          }
          frame "Camera" {
            n162 = call <vilib>:"Get Last Path Segment.vi"("String in"=w322) -> ("String out"=w323:string)  [unwired: 10 in]
            n163 = property on="On/Off" class="Bool (strict)"("Visible"=FALSE) -> ()  [unwired: 2 in, 2 out]
            n164 = property on="Motor" class="Clust (strict)"("Visible"=FALSE) -> ()  [unwired: 2 in, 2 out]
            n165 = property on="Rev/Fwd" class="Clust (strict)"("Visible"=FALSE) -> ()  [unwired: 2 in, 2 out]
            n166 = case shown="\"White Balance  **\"" w323 {
              tunnel: w322 -> [w329 w338 w347 w356 w365 _ w371]
              tunnel: w321 -> [w327 w335 w344 w353 w362 _ _]
              frame "Size  **" {
                n167 = Index Array(array=w327) -> (element=w326:cluster{string[]})  [unwired: 1 in]
                n168 = call <vilib>:"NT Read String.vi"("Name"=w329) -> ("String"=w328:string)  [unwired: 9 in, 1 out]
                n169 = Unbundle(w326) -> (w324:string[])
                n170 = Match First String(2:w324, 3:w328) -> (0:w325:i32)  [unwired: 1 out]
                n171 = property on="Test Ring" class="Ring (strict)"("Value"=w325, "Strings []"=w324) -> ()  [unwired: 2 in, 2 out]
                n172 = property on="Test Ring" class="Ring (strict)"("Visible"=TRUE) -> ()  [unwired: 2 in, 2 out]
                n173 = property on="Test Slider" class="Slide (strict)"("Visible"=FALSE) -> ()  [unwired: 2 in, 2 out]
              }
              frame "White Balance  **" {
                n174 = Index Array(array=w335, index=1) -> (element=w336:cluster{string[]})
                n175 = call <vilib>:"NT Read String.vi"("Name"=w338) -> ("String"=w337:string)  [unwired: 9 in, 1 out]
                n176 = Unbundle(w336) -> (w333:string[])
                n177 = Match First String(2:w333, 3:w337) -> (0:w332:i32)  [unwired: 1 out]
                n178 = property on="Test Ring" class="Ring (strict)"("Value"=w332, "Strings []"=w333) -> ()  [unwired: 2 in, 2 out]
                n179 = property on="Test Ring" class="Ring (strict)"("Visible"=TRUE) -> ()  [unwired: 2 in, 2 out]
                n180 = property on="Test Slider" class="Slide (strict)"("Visible"=FALSE) -> ()  [unwired: 2 in, 2 out]
              }
              frame "Exposure  **" {
                n181 = Index Array(array=w344, index=2) -> (element=w345:cluster{string[]})
                n182 = call <vilib>:"NT Read String.vi"("Name"=w347) -> ("String"=w346:string)  [unwired: 9 in, 1 out]
                n183 = Unbundle(w345) -> (w341:string[])
                n184 = Match First String(2:w341, 3:w346) -> (0:w342:i32)  [unwired: 1 out]
                n185 = property on="Test Ring" class="Ring (strict)"("Value"=w342, "Strings []"=w341) -> ()  [unwired: 2 in, 2 out]
                n186 = property on="Test Ring" class="Ring (strict)"("Visible"=TRUE) -> ()  [unwired: 2 in, 2 out]
                n187 = property on="Test Slider" class="Slide (strict)"("Visible"=FALSE) -> ()  [unwired: 2 in, 2 out]
              }
              frame "Exposure Priority  **" {
                n188 = Index Array(array=w353, index=3) -> (element=w354:cluster{string[]})
                n189 = call <vilib>:"NT Read String.vi"("Name"=w356) -> ("String"=w355:string)  [unwired: 9 in, 1 out]
                n190 = Unbundle(w354) -> (w350:string[])
                n191 = Match First String(2:w350, 3:w355) -> (0:w351:i32)  [unwired: 1 out]
                n192 = property on="Test Ring" class="Ring (strict)"("Value"=w351, "Strings []"=w350) -> ()  [unwired: 2 in, 2 out]
                n193 = property on="Test Ring" class="Ring (strict)"("Visible"=TRUE) -> ()  [unwired: 2 in, 2 out]
                n194 = property on="Test Slider" class="Slide (strict)"("Visible"=FALSE) -> ()  [unwired: 2 in, 2 out]
              }
              frame "Color Enable  **" {
                n195 = Index Array(array=w362, index=4) -> (element=w363:cluster{string[]})
                n196 = call <vilib>:"NT Read String.vi"("Name"=w365) -> ("String"=w364:string)  [unwired: 9 in, 1 out]
                n197 = Unbundle(w363) -> (w359:string[])
                n198 = Match First String(2:w359, 3:w364) -> (0:w360:i32)  [unwired: 1 out]
                n199 = property on="Test Ring" class="Ring (strict)"("Value"=w360, "Strings []"=w359) -> ()  [unwired: 2 in, 2 out]
                n200 = property on="Test Ring" class="Ring (strict)"("Visible"=TRUE) -> ()  [unwired: 2 in, 2 out]
                n201 = property on="Test Slider" class="Slide (strict)"("Visible"=FALSE) -> ()  [unwired: 2 in, 2 out]
              }
              frame Default {
                n202 = property on="Test Ring" class="Ring (strict)"("Visible"=FALSE) -> ()  [unwired: 2 in, 2 out]
                n203 = property on="Test Slider" class="Slide (strict)"("Visible"=FALSE) -> ()  [unwired: 2 in, 2 out]
              }
              frame "Brightness  **", "Color Level  **", "Compression  **", "FPS  **", "Sharpness  **" {
                n204 = call <vilib>:"NT Read Number.vi"("Name"=w371) -> ("Numeric"=w370:dbl)  [unwired: 9 in, 1 out]
                n205 = local write "Test Slider"(w370) -> ()
                n206 = property on="Test Slider" class="Slide (strict)"("Visible"=TRUE, "Scale.Maximum"=100.0 ("Scale.Range:Maximum")) -> ()  [unwired: 2 in, 2 out]
                n207 = property on="Test Ring" class="Ring (strict)"("Visible"=FALSE) -> ()  [unwired: 2 in, 2 out]
              }
            }
          }
        }
        n208 = property on="Progress" class="Clust (strict)"("Visible"=FALSE) -> ()  [unwired: 2 in, 2 out]
      }
      event "Test Name": Mouse Enter {
        # "Populate the ring with the list of tests"
        n209 = event-data() -> ()  [unwired: 1 in, 1 out]
        n210 = call <vilib>:"NT Read String Array.vi"("Name"="/TestMode/TestList") -> ("String Array"=w380:string[])  [unwired: 9 in, 1 out]
        n211 = Build Array (concatenate)("Select the test to run...", w380) -> (w379:string[])
        n212 = property on="Test Name" class="Ring (strict)"("Strings []"=w379) -> ()  [unwired: 2 in, 2 out]
      }
      event "Test Name": Value Change {
        w383 = FALSE ("Visible")
        # "Tell the robot the test name to run"
        n213 = event-data() -> ("NewVal"=w387:u16)  [unwired: 1 in]
        n214 = property on="Test Name" class="Ring (strict)"() -> ("Strings []"=w388:string[])  [unwired: 2 in, 2 out]
        n215 = local write "Progress"(T2 {"Test Progress"=0, "Test Progress Text"=""} ("Progress")) -> ()
        n216 = Index Array(array=w388, index=w387) -> (element=w386:string)
        n217 = call <vilib>:"NT Write String.vi"("String"=w386, "Name"="/TestMode/TestName") -> ()  [unwired: 9 in, 1 out]
        n218 = property on="Progress" class="Clust (strict)"("Visible"=TRUE) -> ()  [unwired: 2 in, 2 out]
        n219 = property on="Motor" class="Clust (strict)"("Visible"=w383) -> ()  [unwired: 2 in, 2 out]
        n220 = property on="Test Slider" class="Slide (strict)"("Visible"=w383) -> ()  [unwired: 2 in, 2 out]
        n221 = property on="On/Off" class="Bool (strict)"("Visible"=w383) -> ()  [unwired: 2 in, 2 out]
        n222 = property on="Rev/Fwd" class="Clust (strict)"("Visible"=w383) -> ()  [unwired: 2 in, 2 out]
        n223 = property on="Test Ring" class="Ring (strict)"("Visible"=w383) -> ()  [unwired: 2 in, 2 out]
      }
      event "Command Selection": Value Change {
        # "Get the params and show in table"
        n224 = event-data() -> ("NewVal"=w393:i32)  [unwired: 1 in]
        n225 = property on="Command Selection" class="MCListbox (strict)"() -> ("ItemNames"=w391:string[][])  [unwired: 2 in, 2 out]
        n226 = call <vilib>:"WPI_DashboardUpdate Command Params.vi"("NewVal"=w393, "Commands"=w391, "Param Tbl"=w392) -> ()  [unwired: 8 in, 1 out]
      }
      event "Execute Command": Value Change {
        # "Started one, Unique ID holds\nresponse"
        n227 = event-data() -> ()  [unwired: 1 in, 1 out]
        n228 = property on="Command Selection" class="MCListbox (strict)"() -> ("ItemNames"=w405:string[][])  [unwired: 2 in, 2 out]
        n229 = Index Array(array=w405, index (row)="Command Selection", index (col)=0) -> (element=w403:string)
        n230 = call <vilib>:"Invoke Commands.vi"("Command Params"="Command Params", "Function Name"=w403) -> ("Params"=w399:u8, "Started"=w398:bool)  [unwired: 7 in, 1 out]
        n231 = Array Subset(array="Command Params", length (row)=w399) -> (w400:string[][])  [unwired: 3 in]
        n232 = Select(t="Executing" ("Cmd Status"), s=w398, f="" ("Cmd Status")) -> (s? t:f=→"Cmd Status":string)
      }
      event "Command Selection": Double Click {
        n233 = event-data() -> ("Row"=w415:i32)  [unwired: 1 in]
        n234 = property on="Command Selection" class="MCListbox (strict)"() -> ("ItemNames"=w418:string[][])  [unwired: 2 in, 2 out]
        n235 = local read "Command Params"() -> (w413:string[][])
        n236 = Index Array(array=w418, index (row)=w415, index (col)=0) -> (element=w416:string)
        n237 = call <vilib>:"Invoke Commands.vi"("Command Params"=w413, "Function Name"=w416) -> ("Params"=w412:u8, "Started"=w407:bool)  [unwired: 7 in, 1 out]
        n238 = Array Subset(array=w413, length (row)=w412) -> (w411:string[][])  [unwired: 3 in]
        n239 = Select(t="Executing" ("Cmd Status"), s=w407, f="" ("Cmd Status")) -> (s? t:f=w408:string)
        n240 = local write "Cmd Status"(w408) -> ()
      }
      event "CheckList": Double Click {
        # "Shift clears all"
        # "Update symbols on the listbox"
        n241 = event-data() -> ("PlatMods.Shift"=w421:bool, "Row"=w423:i32)  [unwired: 1 in]
        n242 = case shown="False" w421 {
          tunnel: w423 -> [w427 _]
          tunnel: 1 -> [w426 _]
          frame False {
            n243 = property on="CheckList" class="LstBox (strict)"() -> ("Item Symbols"=w425:i32[])  [unwired: 2 in, 2 out]
            n244 = Replace Array Subset(array=w425, new element=w426, index=w427) -> (w424:i32[])
            n245 = property on="CheckList" class="LstBox (strict)"("Item Symbols"=w424) -> ()  [unwired: 2 in, 2 out]
          }
          frame True {
            w428 = 0 ("Top Row")
            n246 = property on="CheckList" class="LstBox (strict)"() -> ("Number of Rows"=w430:u32)  [unwired: 2 in, 2 out]
            n247 = Initialize Array(0, w430) -> (w429:i32[])
            n248 = property on="CheckList" class="LstBox (strict)"("Top Row"=w428, "Value"=w428, "Item Symbols"=w429) -> ()  [unwired: 2 in, 2 out]
          }
        }
      }
      event "CheckList": Key Down {
        # "Update symbols on the listbox\nLeft and right keys check and uncheck"
        n249 = event-data() -> ("VKey"=w435:T18)  [unwired: 1 in]
        n250 = case shown="\"Left\", \"Right\"" w435 {
          selector: w435 -> [w440 _]
          tunnel: eventvkey."Left" ("VKey") -> [w438 _]
          frame "Left", "Right" {
            n251 = Equal?(x=w438, y=w440) -> (x = y?=w439:bool)
            n252 = Select(t=0, s=w439, f=1) -> (s? t:f=w441:i32)
            n253 = property on="CheckList" class="LstBox (strict)"() -> ("Item Symbols"=w444:i32[])  [unwired: 2 in, 2 out]
            n254 = Replace Array Subset(array=w444, new element=w441, index="CheckList") -> (w443:i32[])
            n255 = property on="CheckList" class="LstBox (strict)"("Item Symbols"=w443) -> ()  [unwired: 2 in, 2 out]
          }
          frame Default {
          }
        }
      }
      event "DB Camera Config": Value Change {
        # "Show or hide the cluster of controls, store in ini file"
        n256 = event-data() -> ("NewVal"=w449:bool)  [unwired: 1 in]
        n257 = case shown="False" w449 {
          tunnel: w448 -> [w458 _]
          tunnel: [w451 w469] -> w447
          tunnel: w446 -> [w450 w469]
          frame False {
            w465 = "Camera"
            w468 = FALSE ("Visible")
            n258 = local read "Camera Settings"() -> (w457:T6)
            n259 = Index Array(array=w458) -> (element=w461:cluster{string[]})  [unwired: 1 in]
            n260 = Unbundle(w457) -> ("Frame Rate"=w456:i32, "Compression"=w455:i32, "Size"=w459:u16)
            n261 = Unbundle(w461) -> (w460:string[])
            n262 = Index Array(array=w460, index=w459) -> (element=w454:string)
            n263 = call-poly <vilib>:"Write Key.vi"("section"=w465, "value"=w454, "key"="Size", "refnum"=w450) -> ("refnum out"=w467:T12)  [unwired: 2 in, 5 out]
            n264 = call-poly <vilib>:"Write Key.vi"("section"=w465, "value"=w456, "key"="FrameRate", "refnum"=w467) -> ("refnum out"=w466:T12)  [unwired: 1 in, 6 out]
            n265 = property on="Camera Settings" class="Clust (strict)"("Visible"=w468) -> ()  [unwired: 2 in, 2 out]
            n266 = local write "DB Camera Config"(w468) -> ()
            n267 = call-poly <vilib>:"Write Key.vi"("section"=w465, "value"=w455, "key"="Compression", "refnum"=w466) -> ("refnum out"=w452:T12)  [unwired: 1 in, 6 out]
            n268 = call <vilib>:"Close Config Data.vi"("refnum"=w452) -> ("file path"=w453:path)  [unwired: 2 in, 8 out]
            n269 = call <vilib>:"Open Config Data.vi"("configuration file path"=w453) -> ("refnum"=w451:T12)  [unwired: 8 in, 2 out]
          }
          frame True {
            n270 = property on="Camera Settings" class="Clust (strict)"("Visible"=TRUE) -> ()  [unwired: 2 in, 2 out]
          }
        }
      }
      event "Camera Settings": Value Change {
        # "Update summary string when any elements of DB camera change"
        n271 = event-data() -> ("NewVal"=w483:T6)  [unwired: 1 in]
        n272 = Index Array(array=w479) -> (element=w478:cluster{string[]})  [unwired: 1 in]
        n273 = Unbundle(w483) -> ("Frame Rate"=w474:i32, "Compression"=w473:i32, "Size"=w476:u16)
        n274 = Unbundle(w478) -> (w477:string[])
        n275 = Index Array(array=w477, index=w476) -> (element=w475:string)
        n276 = Format Into String(format string="%s   %dfps   %d%%", w475, w474, w473) -> (resulting string=w480:string)  [unwired: 2 in, 1 out]
        n277 = Build Array(w480) -> (w481:string[])
        n278 = property on="DB Camera Config" class="Bool (strict)"("Strings [4]"=w481) -> ()  [unwired: 2 in, 2 out]
      }
      event "Motor.Enable": Value Change {
        # "When the test mode otor enable helper is set, update that\ntree row item's value"
        n279 = event-data() -> ("NewVal"=w490:bool)  [unwired: 1 in]
        n280 = Unbundle("Motor") -> ("Value"=w489:dbl)  [unwired: 1 out]
        n281 = Select(t=w489, s=w490, f=0.0) -> (s? t:f=w487:dbl)
        n282 = call <vilib>:"NT Write Number.vi"("Numeric"=w487, "Name"=w486) -> ()  [unwired: 9 in, 1 out]
      }
      event "Test Slider": Value Change {
        # "When the test mode slider helper is set, update that\ntree row item's value"
        n283 = event-data() -> ("NewVal"=w494:dbl)  [unwired: 1 in]
        n284 = call <vilib>:"NT Write Number.vi"("Numeric"=w494, "Name"=w495) -> ()  [unwired: 9 in, 1 out]
      }
      event "On/Off": Value Change {
        # "When the test mode on/off helper value is set, update that\ntree row item's value"
        n285 = event-data() -> ("NewVal"=w500:bool)  [unwired: 1 in]
        n286 = Boolean To (0,1)(Boolean=w500) -> (0, 1=w499:i16)
        n287 = call <vilib>:"NT Write Number.vi"("Numeric"=w499, "Name"=w498) -> ()  [unwired: 9 in, 1 out]
      }
      event "Rev/Fwd": Value Change {
        # "When the test mode helper value for relays is set, update that\ntree row item's value"
        n288 = event-data() -> ("NewVal.Forward"=w509:bool, "NewVal.Reverse"=w508:bool)  [unwired: 1 in]
        n289 = Boolean To (0,1)(Boolean=w509) -> (0, 1=w505:i16)
        n290 = Boolean To (0,1)(Boolean=w508) -> (0, 1=w507:i16)
        n291 = Negate(x=w507) -> (-x=w506:i16)
        n292 = Add(x=w505, y=w506) -> (x+y=w504:i16)
        n293 = call <vilib>:"NT Write Number.vi"("Numeric"=w504, "Name"=w503) -> ()  [unwired: 9 in, 1 out]
      }
      event "Test Ring": Value Change {
        # "When a test mode helper value is selected from the ring,\nset the tree item's variable to the string value"
        n294 = event-data() -> ("NewVal"=w514:u16)  [unwired: 1 in]
        n295 = property on="Test Ring" class="Ring (strict)"() -> ("Strings []"=w515:string[])  [unwired: 2 in, 2 out]
        n296 = Index Array(array=w515, index=w514) -> (element=w513:string)
        n297 = call <vilib>:"NT Write String.vi"("String"=w513, "Name"=w512) -> ()  [unwired: 9 in, 1 out]
      }
      event "Rec Mode": Value Change {
        # "Update globals for recording mode and path to read log from.\nClear when logging and let NetworkTables set path for vision to\nuse."
        n298 = event-data() -> ("NewVal"=w527:enum32{"Stop", "Record", "Playback"})  [unwired: 1 in]
        n299 = global write "WPI_DashboardLogging Global.vi" "Logging Filename"(path "") -> ()
        n300 = global write "WPI_DashboardLogging Global.vi" "Recording"(w527) -> ()
        n301 = case shown="\"Playback\"" w527 {
          tunnel: w526 -> [_ w529 w538]
          tunnel: [_ _ w537] -> w523
          tunnel: [_ _ w536] -> _
          tunnel: w521 -> [_ _ w534]
          tunnel: cluster{i32, i32} {-250, 170} -> [_ _ w533]
          tunnel: [_ _ T19 {"Image Size"=TRUE, "Image Type"=TRUE, "Pixel Value"=TRUE, "ROI Information"=TRUE, "Zoom Factor"=FALSE} ("Image Information Shown:All Elements")] -> w519
          tunnel: [_ _ TRUE ("Zoom Factor")] -> w518
          tunnel: w517 -> [_ _ w530]
          frame Default {
          }
          frame "Stop", "Record" {
            # "Place Window too"
            n302 = invoke class="VI" method="FP.Close"(reference=w529) -> (reference out=w528:refnum<vi>)  [unwired: 2 in, 2 out]
            n303 = invoke class="VI" method="Abort VI"(reference=w528) -> ()  [unwired: 2 in, 3 out]
          }
          frame "Playback" {
            n304 = call "Open Playback Panel.vi"("Offset"=w533, "DB VI Ref"=w534, "Playback in"=w538) -> ("Playback out"=w535:refnum<vi>)  [unwired: 8 in]
            n305 = register-events(w535, w530) -> (reference out=w537:refnum<event-registration>, error out=w536:errorcluster)  [unwired: 2 in]
          }
        }
        n306 = property on="Camera Image" class="ImageControl"("Image Information Shown"=w519, "Image Information Visible"=w518) -> ()  [unwired: 2 in, 2 out]
        n307 = call <vilib>:"WPI_DashboardNT Log FieldName Cache.vi"("Operation"=enum16{"Lookup/Add", "Index", "Clear"}."Clear") -> ()  [unwired: 8 in, 3 out]
      }
      event Panel Close {
        w540 = enum32{"Stop", "Record", "Playback"}."Stop" ("Rec Mode")
        # "Playback window has been closed, abort"
        n308 = event-data() -> ()  [unwired: 1 in, 4 out]
        n309 = local write "Rec Mode"(w540) -> ()
        n310 = global write "WPI_DashboardLogging Global.vi" "Recording"(w540) -> ()
      }
      event Panel Close {
        # "Abort playback window and ourself"
        n311 = event-data() -> ()  [unwired: 1 in, 4 out]
        n312 = invoke class="VI" method="FP.Close"(reference=w546) -> (reference out=w545:refnum<vi>)  [unwired: 2 in, 2 out]
        n313 = invoke class="VI" method="Abort VI"(reference=w545) -> (error out=w544:errorcluster)  [unwired: 2 in, 2 out]
        n314 = invoke class="VI" method="Abort VI"(error in=w544) -> ()  [unwired: 2 in, 3 out]
      }
      event User Event {
        n315 = event-data() -> ("IDs"=w554:cluster{"RPC field ID":u16, "Unique ID":u16}, "String"=w553:string)  [unwired: 1 in]
        n316 = Bundle("IDs"=w554, "String"=w553) -> (w552:T10)  [unwired: 1 in]
        n317 = call <vilib>:"Retrieve RPC Response.vi"("RPC Response"=w552) -> ("Output"=w549:string[][])  [unwired: 10 in]
        n318 = Build Array (concatenate)(w547, w549) -> (w548:string[][])
        n319 = local write "Command Params"(w548) -> ()
        n320 = local write "Cmd Status"("" ("Cmd Status")) -> ()
      }
      event "Vision": Value Change {
        # "Enable/Disable Compression slider.\nHW USB is hard-coded into the camera"
        n321 = event-data() -> ("NewVal"=w561:u16)  [unwired: 1 in]
        n322 = Equal?(x=w561, y=u32 2 ("milliseconds to wait")) -> (x = y?=w559:bool)
        n323 = Select(t=T20."Disabled and Grayed Out" ("Disabled"), s=w559, f=T20."Enabled" ("Disabled")) -> (s? t:f=w556:T20)
        n324 = property on="Compression" class="Slide (strict)"("DisabledEnum"=w556) -> ()  [unwired: 2 in, 2 out]
      }
      event "Tree": Double Click {
        n325 = event-data() -> ("PlatMods"=w566:T23, "Tag"=w565:string)  [unwired: 1 in]
        n326 = Unbundle(w566) -> ("Shift"=w564:bool)  [unwired: 4 out]
        n327 = Not(x=w564) -> (.not. x?=w563:bool)
        n328 = call <vilib>:"NT Update Persistence.vi"("Persistence"=w563, "Name"=w565) -> ()  [unwired: 9 in, 1 out]
      }
    }
  }
  n329 = while {
    tunnel: w89 -> [w570]
    i -> [w573]
    stop <- FALSE stop-if-true
    n330 = Wait (ms)(milliseconds to wait=u32 100) -> ()  [unwired: 1 out]
    n331 = case shown="\"Playback\"" "Rec Mode" {
      tunnel: w573 -> [_ _ w588]
      tunnel: [u32 2829099 ("Base Color") u32 11141120 ("Target Color") w577] -> w569
      frame "Stop", Default {
        # "Reset the color, extra updates don't cost much"
      }
      frame "Record" {
      }
      frame "Playback" {
        # "Playback"
        n332 = Quotient & Remainder(x=w588, y=u32 50 ("milliseconds to wait")) -> (x-y*floor(x/y)=w584:u32)  [unwired: 1 out]
        n333 = Divide(x=w584, y=u32 50 ("milliseconds to wait")) -> (x/y=w581:dbl)
        n334 = Multiply(x=6.283185307179586, y=w581) -> (x*y=w586:dbl)
        n335 = Sine(x=w586) -> (sin(x)=w585:dbl)
        n336 = Absolute Value(x=w585) -> (abs(x)=w578:dbl)
        n337 = call "Interpolate RGB Color.vi"("Proportion"=w578, "Target Color"=u32 30976, "Base Color"=u32 2829099) -> ("Result Color"=w577:u32)  [unwired: 8 in]
      }
    }
    n338 = property class="Pane"(reference=w570, "PaneColor"=w569) -> ()  [unwired: 1 in, 2 out]
  }
  n339 = local write "Dashboard Tab"(T1."Drive" ("Dashboard Tab")) -> ()
  n340 = call "Image Process Cal Wright 2016.vi"("Path"=w42) -> ("Settings"=w54:T24)  [unwired: 3 out]
  n341 = Unbundle By Name(w54) -> ("Hue Max"=w45:dbl, "Hue Min"=w46:dbl, "Sat Max"=w47:dbl, "Sat Min"=w48:dbl, "Val Max"=w49:dbl, "Val Min"=w50:dbl, "Far Shot Distance (ft)"=w41:dbl, "Close Shot Distance (ft)"=w40:dbl, "X 1"=w39:dbl, "Y 1"=w38:dbl, "Thickness 1"=w37:dbl, "Input 1"=w36:dbl, "X 2"=w35:dbl, "Y 2"=w34:dbl, "Thickness 2"=w33:dbl, "Input 2"=w32:dbl, "Min Score"=w31:dbl)
  n342 = Bundle("Hue Max"=w45, "Hue Min"=w46) -> (w52:cluster{"Hue Max":dbl, "Hue Min":dbl})  [unwired: 1 in]
  n343 = Bundle("Sat Max"=w47, "Sat Min"=w48) -> (w51:cluster{"Sat Max":dbl, "Sat Min":dbl})  [unwired: 1 in]
  n344 = Bundle("Val Max"=w49, "Val Min"=w50) -> (w53:cluster{"Val Max":dbl, "Val Min":dbl})  [unwired: 1 in]
  n345 = local write "Min Score"(w31) -> ()
  n346 = local write "Far Shot Distance (ft)"(w41) -> ()
  n347 = local write "Close Shot Distance (ft)"(w40) -> ()
  n348 = local write "X 1"(w39) -> ()
  n349 = local write "Y 1"(w38) -> ()
  n350 = local write "Thickness 1"(w37) -> ()
  n351 = local write "X 2"(w35) -> ()
  n352 = local write "Y 2"(w34) -> ()
  n353 = local write "Thickness 2"(w33) -> ()
  n354 = local write "Input 1"(w36) -> ()
  n355 = local write "Input 2"(w32) -> ()
  n356 = Bundle By Name(cluster=T4 {"Hue"={110.0, 142.0}, "Sat"={138.0, 255.0}, "Val"={139.0, 198.0}} ("Color Components"), "Hue"=w52, "Sat"=w51, "Val"=w53) -> (w44:T4)
  n357 = local write "Reflective Tape Color"(w44) -> ()
  n358 = call "IMAQ Create"("Image Name"="Mask", "Image Type"=w68) -> ("New Image"=w67:T8)  [unwired: 2 in, 2 out]
  n359 = while {
    tunnel: w65 -> [w605]
    tunnel: [w606] -> _
    tunnel: w67 -> [w597]
    tunnel: w55 -> [w593]
    tunnel: w42 -> [w592]
    i -> [w606]
    stop <- FALSE stop-if-true
    n360 = local read "Rec Mode"() -> (w600:enum32{"Stop", "Record", "Playback"})
    n361 = local read "Camera IP"() -> (w594:string)
    n362 = Not Equal?(x="Vision", y=u16 4) -> (x != y?=w591:bool)
    n363 = case shown="False" w591 {
      tunnel: w605 -> [w614 w623]
      tunnel: [w610 w622] -> w604
      tunnel: [TRUE ("Active") w621] -> w603
      tunnel: [0.0 ("FPS") w620] -> w602
      tunnel: "Camera Settings" -> [w613 w619]
      tunnel: w600 -> [_ w618]
      tunnel: "Vision" -> [_ w617]
      tunnel: [0.0 ("Bandwidth (Mbps)") w616] -> w599
      tunnel: w594 -> [_ w615]
      frame False {
        n364 = call <vilib>:"WPI_CameraDirect Read from Laptop.vi"("Camera Settings"=w613, "Image"=w614, "address"="USB 2") -> ("Image Out"=w610:T8)  [unwired: 7 in, 1 out]
      }
      frame True {
        n365 = call <vilib>:"WPI_CameraRead MJPG for Dashboard.vi"("Camera Settings"=w619, "Rec Mode"=w618, "Camera IP"=w615, "Camera Mode"=w617, "Refnum in"=w623) -> ("Active"=w621:bool, "Refnum out"=w622:T8, "FPS"=w620:dbl, "Bandwidth (Mbps)"=w616:dbl)  [unwired: 3 in]
      }
    }
    "Mbps" <- w599
    n366 = Or(x=w603, y="Test Mode") -> (x .or. y?=w598:bool)
    n367 = Not(x="Test Mode") -> (.not. x?=w596:bool)
    n368 = case shown="True" w598 {
      tunnel: w604 -> [_ w681]
      tunnel: w599 -> [_ w682]
      tunnel: w602 -> [_ w680]
      tunnel: w596 -> [_ w679]
      tunnel: w597 -> [_ w678]
      tunnel: w593 -> [_ w664]
      tunnel: w592 -> [_ w651]
      frame False {
        w624 = u32 1985280 ("Color Box")
        # "Test Mode off and no camera signal"
        # "Sleep for 500ms"
        n369 = Bundle("Color Box"=w624, "Color Box"=w624) -> (w626:cluster{"Color Box":u32, "Color Box":u32})  [unwired: 1 out]
        n370 = Build Array(w626) -> (w625:cluster{"Color Box":u32, "Color Box":u32}[])
        n371 = property on="Mbps LED" class="Bool (strict)"("Colors [4]"=w625) -> ()  [unwired: 2 in, 2 out]
        n372 = Wait Until Next ms Multiple(millisecond multiple=u32 500) -> ()  [unwired: 1 out]
      }
      frame True {
        # "TODO: draw distance under target box"
        # "Overlay crosshairs"
        # "Calculate crosshair position by simply clicking on the image"
        # "Draw target box"
        # "Generate target data from image"
        # "Allow the user to change HSV values by drawing \nlines over the image\n-- Disabled due to lag"
        # "Use a test image or the camera stream depending on Test Mode"
        n373 = case shown="True" w679 {
          tunnel: w681 -> [_ w754]
          tunnel: w682 -> [_ w757]
          tunnel: [w749 w754] -> w631
          tunnel: w680 -> [_ w756]
          tunnel: w664 -> [w750 _]
          frame False {
            w752 = u32 1985280 ("Color Box")
            n374 = Bundle("Color Box"=w752, "Color Box"=w752) -> (w753:cluster{"Color Box":u32, "Color Box":u32})  [unwired: 1 out]
            n375 = Build Array(w753) -> (w751:cluster{"Color Box":u32, "Color Box":u32}[])
            n376 = call "IMAQ Clear Overlay"("Image"=w750) -> ("Image Out"=w749:T8)  [unwired: 9 in, 1 out]
            n377 = property on="Mbps LED" class="Bool (strict)"("Colors [4]"=w751) -> ()  [unwired: 2 in, 2 out]
          }
          frame True {
            # "Update Mbps LED"
            n378 = case shown="Default" w757 {
              tunnel: [u32 6618880 ("Color Box") u32 16776722 ("Color Box") u32 16716800 ("Color Box")] -> w758
              frame Default {
              }
              frame 4, 5 {
              }
              frame 6.. {
              }
            }
            n379 = Bundle("Color Box"=w758, "Color Box"=w758) -> (w759:cluster{"Color Box":u32, "Color Box":u32})  [unwired: 1 out]
            n380 = Build Array(w759) -> (w755:cluster{"Color Box":u32, "Color Box":u32}[])
            n381 = property on="Mbps LED" class="Bool (strict)"("Colors [4]"=w755) -> ()  [unwired: 2 in, 2 out]
            "fps" <- w756
          }
        }
        n382 = local read "Reflective Tape Color"() -> (w658:T4)
        n383 = local read "Close Shot Distance (ft)"() -> (w647:dbl)
        n384 = local read "Far Shot Distance (ft)"() -> (w648:dbl)
        n385 = local read "Thickness 1"() -> (w644:dbl)
        n386 = local read "Thickness 2"() -> (w640:dbl)
        n387 = local read "Min Score"() -> (w638:dbl)
        n388 = local read "Input 1"() -> (w643:u32)
        n389 = local read "Input 2"() -> (w639:u32)
        n390 = Unbundle By Name(w658) -> ("Hue"=w660:cluster{dbl, dbl}, "Sat"=w661:cluster{dbl, dbl}, "Val"=w659:cluster{dbl, dbl})
        n391 = local read "X 1"() -> (w646:dbl)
        n392 = local read "Y 1"() -> (w645:dbl)
        n393 = local read "X 2"() -> (w642:dbl)
        n394 = local read "Y 2"() -> (w641:dbl)
        n395 = Unbundle(w660) -> (w656:dbl, w657:dbl)
        n396 = Unbundle(w661) -> (w655:dbl, w654:dbl)
        n397 = Unbundle(w659) -> (w653:dbl, w652:dbl)
        n398 = disable-structure shown="Enabled" {
          disable-tunnel: w631 -> [w688 _]
          frame Enabled {
            n399 = case shown="True" "Calibrate" {
              tunnel: w688 -> [_ w689]
              frame False {
              }
              frame True {
                w691 = u16 2 items=["RGB", "HSL", "HSV", "HSI", "CIE L*a*b*", "CIE XYZ"] ("Color Mode")
                # "Standard Deviations"
                n400 = control-ref of="Camera Image"() -> (w694:refnum<vi>)
                n401 = call "Calibration Helper2.vi"("Std Devs"=cluster{"H":dbl, "S":dbl, "V":dbl} {"H"=4.0, "S"=6.0, "V"=6.0}, "Color Mode"=w691, "Color Components"="Reflective Tape Color", "Image"=w689, "Image Ctl Refnum"=w694) -> ("Changed"=w690:bool, "output color"=w692:T25)  [unwired: 5 in]
                n402 = case shown="True" w690 {
                  tunnel: w692 -> [_ w696]
                  frame False {
                  }
                  frame True {
                    n403 = local write "Reflective Tape Color"(w696) -> ()
                  }
                }
              }
            }
          }
          frame Disabled {
          }
        }
        n404 = Bundle(w656, w657, w655, w654, w653, w652, "Far Shot Distance (ft)"=w648, "Close Shot Distance (ft)"=w647, "X 1"=w646, "Y 1"=w645, "Thickness 1"=w644, "Input 1"=w643, "X 2"=w642, "Y 2"=w641, "Thickness 2"=w640, "Input 2"=w639, "Min Score"=w638) -> (w650:T26)  [unwired: 1 in]
        n405 = call "Image Process Cal Read 2016.vi"("Path"=w651, "PreSET Save"=TRUE, "Input cluster"=w650, "Save Values"="Save Settings") -> ("file created?"=w636:bool)  [unwired: 1 in]
        "File Created" <- w636
        n406 = Select(t="Saved", s=w636, f="") -> (s? t:f=→"Status":string)
        n407 = local read "Reflective Tape Color"() -> (w676:T4)
        n408 = call "Recognize Goal.vi"("Camera Type"="Camera", "HSV"=w676, "Min Score Threshold"="Min Score", "Image Dst"=w678, "Image In"=w631) -> ("Highest Average Score"=w666:dbl, "Target With Highest Average Score"=w671:T27, "All Targets Found"=w672:T28)  [unwired: 2 in]
        "Highest Score" <- w666
        n409 = Array Size(array=w672) -> (size(s)=→"Targets":i32)
        n410 = Greater Or Equal?(x=w666, y="Min Score") -> (x >= y?=w665:bool)
        n411 = call "Denormalize Target.vi"("Target In"=w671, "Image In"=w678) -> ("Target Out"=w673:T29)  [unwired: 9 in]
        n412 = local write "Target Indicator"(w665) -> ()
        n413 = Unbundle By Name(w673) -> ("Distance (ft)"=w629:dbl, "Center"=w668:cluster{dbl, dbl}, "Bounding Rect"=w632:T30)
        "Distance (ft)" <- w629
        "Distance" <- w629
        n414 = disable-structure shown="Disabled" {
          disable-tunnel: w631 -> [w686 _]
          disable-tunnel: [w683 _] -> _
          frame Disabled {
            n415 = call "IMAQ GetImageSize"("Image"=w686) -> ("X Resolution"=w685:i32)  [unwired: 3 in, 2 out]
            n416 = Divide(x=w685, y=2) -> (x/y=w683:dbl)
          }
          frame Enabled {
          }
        }
        n417 = Unbundle(w668) -> (→"Vision Target Center" →"Target Align Center":dbl)  [unwired: 1 out]
        n418 = call-poly <vilib>:"NT Write Value.vi"("Numeric"=w629, "Name"="Distance") -> ()  [unwired: 9 in, 1 out]
        n419 = local read "X 1"() -> (→"Robot Center":dbl)
        n420 = case shown="True" "Show Target Box" {
          tunnel: w631 -> [w712 w726]
          tunnel: w632 -> [_ w725]
          tunnel: w668 -> [_ w715]
          tunnel: [w712 w714] -> w663
          frame False {
          }
          frame True {
            w722 = u32 0 items=["Frame", "Fill", "Highlight"] ("Drawing Mode (Frame)")
            # "Change color of box depending on distance"
            n421 = local read "Distance (ft)"() -> (w723:dbl)
            n422 = Less Or Equal?(x=w723, y="Far Shot Distance (ft)") -> (x <= y?=w713:bool)
            n423 = local write "Distance Indicator"(w713) -> ()
            n424 = case shown="True" w713 {
              tunnel: w723 -> [_ w746]
              tunnel: ["Too Far" w743] -> w716
              frame False {
              }
              frame True {
                n425 = Less Or Equal?(x=w746, y="Close Shot Distance (ft)") -> (x <= y?=w744:bool)
                n426 = case shown="True" w744 {
                  tunnel: ["Far Shot" "Close Shot"] -> w743
                  frame False {
                  }
                  frame True {
                  }
                }
              }
            }
            n427 = call "IMAQ Overlay Rectangle"("Color"=w716, "Drawing Mode (Frame)"=w722, "Rectangle"=w725, "Image"=w726) -> ("Image Out"=w721:T8)  [unwired: 6 in, 1 out]
            n428 = call "Overlay Crosshairs.vi"("Image In"=w721, "Coordinates"=w715, "Crosshair Length (px)"=10.0, "Crosshair Thickness"=2.0, "Color"=w716) -> ("Image Out"=w717:T8)  [unwired: 4 in]
            n429 = case shown="False" "Show Center Line" {
              tunnel: w717 -> [w727 w740]
              tunnel: w716 -> [_ w733]
              tunnel: w715 -> [_ w741]
              tunnel: [w727 w729] -> w714
              frame False {
              }
              frame True {
                w732 = 1 ("Thickness")
                w734 = 500
                w736 = 0
                n430 = Unbundle(w741) -> (w738:dbl)  [unwired: 1 out]
                n431 = Bundle(w738, w734) -> (w739:cluster{dbl, i32})  [unwired: 1 in]
                n432 = Bundle(w738, w736) -> (w737:cluster{dbl, i32})  [unwired: 1 in]
                n433 = call "Line ovelay one.vi"("Thickness"=w732, "Color"=w733, "End Point"=w737, "Start Point"=w739, "Image"=w740) -> ("Image Out"=w728:T8)  [unwired: 5 in, 1 out]
                n434 = local read "Robot Center"() -> (w735:dbl)
                n435 = Bundle("Robot Center"=w735, w734) -> (w730:cluster{"Robot Center":dbl, i32})  [unwired: 1 in]
                n436 = Bundle("Robot Center"=w735, w736) -> (w731:cluster{"Robot Center":dbl, i32})  [unwired: 1 in]
                n437 = call "Line ovelay one.vi"("Thickness"=w732, "Color"=w733, "End Point"=w731, "Start Point"=w730, "Image"=w728) -> ("Image Out"=w729:T8)  [unwired: 5 in, 1 out]
              }
            }
          }
        }
        n438 = case shown="True" "Show Crosshairs" {
          tunnel: [w697 w702] -> w677
          tunnel: w663 -> [w697 w701]
          frame False {
          }
          frame True {
            w707 = 700
            # "Far shot crosshair"
            # "Close shot crosshair"
            n439 = Bundle("X 1"="X 1", "Y 1"="Y 1") -> (w709:cluster{"X 1":dbl, "Y 1":dbl})  [unwired: 1 in]
            n440 = call "Overlay Crosshairs.vi"("Image In"=w701, "Coordinates"=w709, "Crosshair Length (px)"=w707, "Crosshair Thickness"="Thickness 1", "Color"=u32 524468) -> ("Image Out"=w703:T8)  [unwired: 4 in]
            n441 = Bundle("X 2"="X 2", "Y 2"="Y 2") -> (w700:cluster{"X 2":dbl, "Y 2":dbl})  [unwired: 1 in]
            n442 = call "Overlay Crosshairs.vi"("Image In"=w703, "Coordinates"=w700, "Crosshair Length (px)"=w707, "Crosshair Thickness"="Thickness 2", "Color"=u32 16769834) -> ("Image Out"=w702:T8)  [unwired: 4 in]
          }
        }
        "Camera Image" <- w677
      }
    }
  }
  n443 = property on="On/Off" class="Bool (strict)"("Visible"=w79) -> ()  [unwired: 2 in, 2 out]
  n444 = property on="Motor" class="Clust (strict)"("Visible"=w79) -> ()  [unwired: 2 in, 2 out]
  n445 = property on="Progress" class="Clust (strict)"("Visible"=w79) -> ()  [unwired: 2 in, 2 out]
  n446 = property on="Test Ring" class="Ring (strict)"("Visible"=w79) -> ()  [unwired: 2 in, 2 out]
  n447 = property on="Rev/Fwd" class="Clust (strict)"("Visible"=w79) -> ()  [unwired: 2 in, 2 out]
  n448 = property on="Camera Settings" class="Clust (strict)"("Visible"=w79) -> ()  [unwired: 2 in, 2 out]
  n449 = local write "DB Camera Config"(w79) -> ()
  n450 = local write "Command Params"(string[][] [] ("Command Params")) -> ()
  n451 = global write "WPI_DashboardLogging Global.vi" "Recording"(w84) -> ()
  n452 = local write "Rec Mode"(w84) -> ()
  n453 = while {
    tunnel: u16 1741 ("timeout ms (25000)") -> [w764]
    stop <- FALSE stop-if-true
    n454 = TCP Create Listener(10:w764) -> (0:w763:errorcluster, 3:w765:refnum<k5>)  [unwired: 4 in, 1 out]
    n455 = case shown="No Error" w763 {
      selector: w763 -> [w767 _]
      tunnel: w765 -> [w768 _]
      frame No Error {
        n456 = while {
          tunnel: w768 -> [w771]
          tunnel: w767 -> [w770]
          stop <- FALSE stop-if-true
          n457 = TCP Wait On Listener(8:w770, 11:w771) -> (0:w772:errorcluster, 4:w773:refnum<k5>)  [unwired: 2 in, 3 out]
          n458 = local write "TCP"(w773) -> ()
          n459 = case shown="No Error" w772 {
            frame No Error {
            }
            frame Error {
              n460 = Wait (ms)(milliseconds to wait=u32 1000) -> ()  [unwired: 1 out]
            }
          }
        }
      }
      frame Error {
        n461 = Wait (ms)(milliseconds to wait=u32 1000) -> ()  [unwired: 1 out]
      }
    }
  }
  n462 = local write "Command Selection"(u16 0 ("milliseconds to wait")) -> ()
  "INI File Path" <- w42
